vi "transfer char run_subvi_SMU4_14_05_22_JWa.vi"(0 "VISA session":refnum<visa-resource-name>="GPIB0::17::INSTR", 1 "Y2 axis settings":T5={"Y2 axis on/off"=FALSE, "MINIMUM"=0.0, "MAXIMUM"=1.0, "Variable name"="Ig", "LIN or LOG axis"="LIN"} {"MAXIMUM" format="%.9f"; "MINIMUM" format="%.9f"}, 3 "LKG Path":path, 5 "Var1 sweep settings":T7={"start"=40.0, "stop"=-40.0, "step (linear only)"=-1.0, "sweep spacing (linear: 0)"=0, "sweep mode"=FALSE, "compliance (V)"=100.0, "compliance (A)"=0.001} {"compliance (A)" format="%^.2e"; "compliance (V)" format="%.2f"; "sweep spacing (linear: 0)" items=["linear", "log 10", "log 25", "log 50"]; "step (linear only)" format="%.2f"; "stop" format="%.2f"; "start" format="%.2f"}, 7 "Var2 step settings":T6={"compliance (A)"=0.001, "compliance (V)"=100.0, "start"=-2.0, "total points"=2, "step"=-38.0} {"step" format="%.2f"; "start" format="%.2f"; "compliance (V)" format="%.2f"; "compliance (A)" format="%^.2e"}, 9 "integration time":u32(slide) scale=0.0..2.0, 11 "Input Path":path, 12 "Dielectric Constant":dbl=5.0, 13 "Sample Properties:":T4 {"Date Created" format="%<%x>T"}) -> (2 "Check Cluster":T2, 4 "Output":T3 {"Mobility-Lin" format="%#_4e"; "Mobility-Sat" format="%#_4e"}, 6 "Graph Cluster":T1, 15 "error?":errorcluster)   [LabVIEW 2012]
uses:
  <vilib>/Utility/file.llb/Write To Spreadsheet File (DBL).vi
panel:
  out "concatenated string":string
  in  "Output Path":path
  in  "Temp (K)":dbl=0.001 format="%^.2e"
  in  "NumPts":dbl=5.0
  out "Numeric":dbl
  out "min r":dbl
  out "max r":dbl
  out "error? 2":errorcluster
  in  "MAXIMUM":ext format="%.2e"
  in  "MINIMUM":ext=-1e-05 format="%_2e"
  out "Gate Current Plot":cluster{"trace":dbl[], "trace":dbl[]}(graph)
  in  "Y1 axis":string="Id"
  out "graphic display":cluster{"trace":dbl[], "trace":dbl[]}(graph)
  in  "wait time parameter":dbl=1.0
  in  "Value (Either V or A) 4":dbl
  in  "Value (Either V or A) 3":dbl
  in  "Value (Either V or A) 2":dbl
  in  "Value (V or A)":dbl
  in  "compliance (A)":dbl=0.001 format="%^.2e"
  in  "compliance (V)":dbl=100.0 format="%^.2e"
  in  "Iname":string="Is"
  in  "Vname":string="Vs"
  in  "Function":u16(ring)=4 items=["disabled", "Var1", "Var2", "Var1'", "Constant"]
  in  "Mode":u16(ring)=4 items=["V", "I", "VPulse", "IPulse", "Common"]
  in  "Iname 4":string="Ig"
  in  "Vname 4":string="Vg"
  in  "Function 4":u16(ring)=1 items=["disabled", "Var1", "Var2", "Var1'", "Constant"]
  in  "Mode 4":u16(ring) items=["V", "I", "VPulse", "IPulse", "Common"]
  in  "Iname 3":string="I3"
  in  "Vname 3":string="V3"
  in  "Function 3":u16(ring)=4 items=["disabled", "Var1", "Var2", "Var1'", "Constant"]
  in  "Mode 3":u16(ring) items=["V", "I", "VPulse", "IPulse", "Common"]
  in  "Iname 2":string="Id"
  in  "Vname 2":string="Vd"
  in  "Function 2":u16(ring)=2 items=["disabled", "Var1", "Var2", "Var1'", "Constant"]
  in  "Mode 2":u16(ring) items=["V", "I", "VPulse", "IPulse", "Common"]
  in  "reset":bool=TRUE
  # "SMU1"
  # "SMU2"
  # "SMU3"
  # "SMU4"
  # "Sample Properties:"
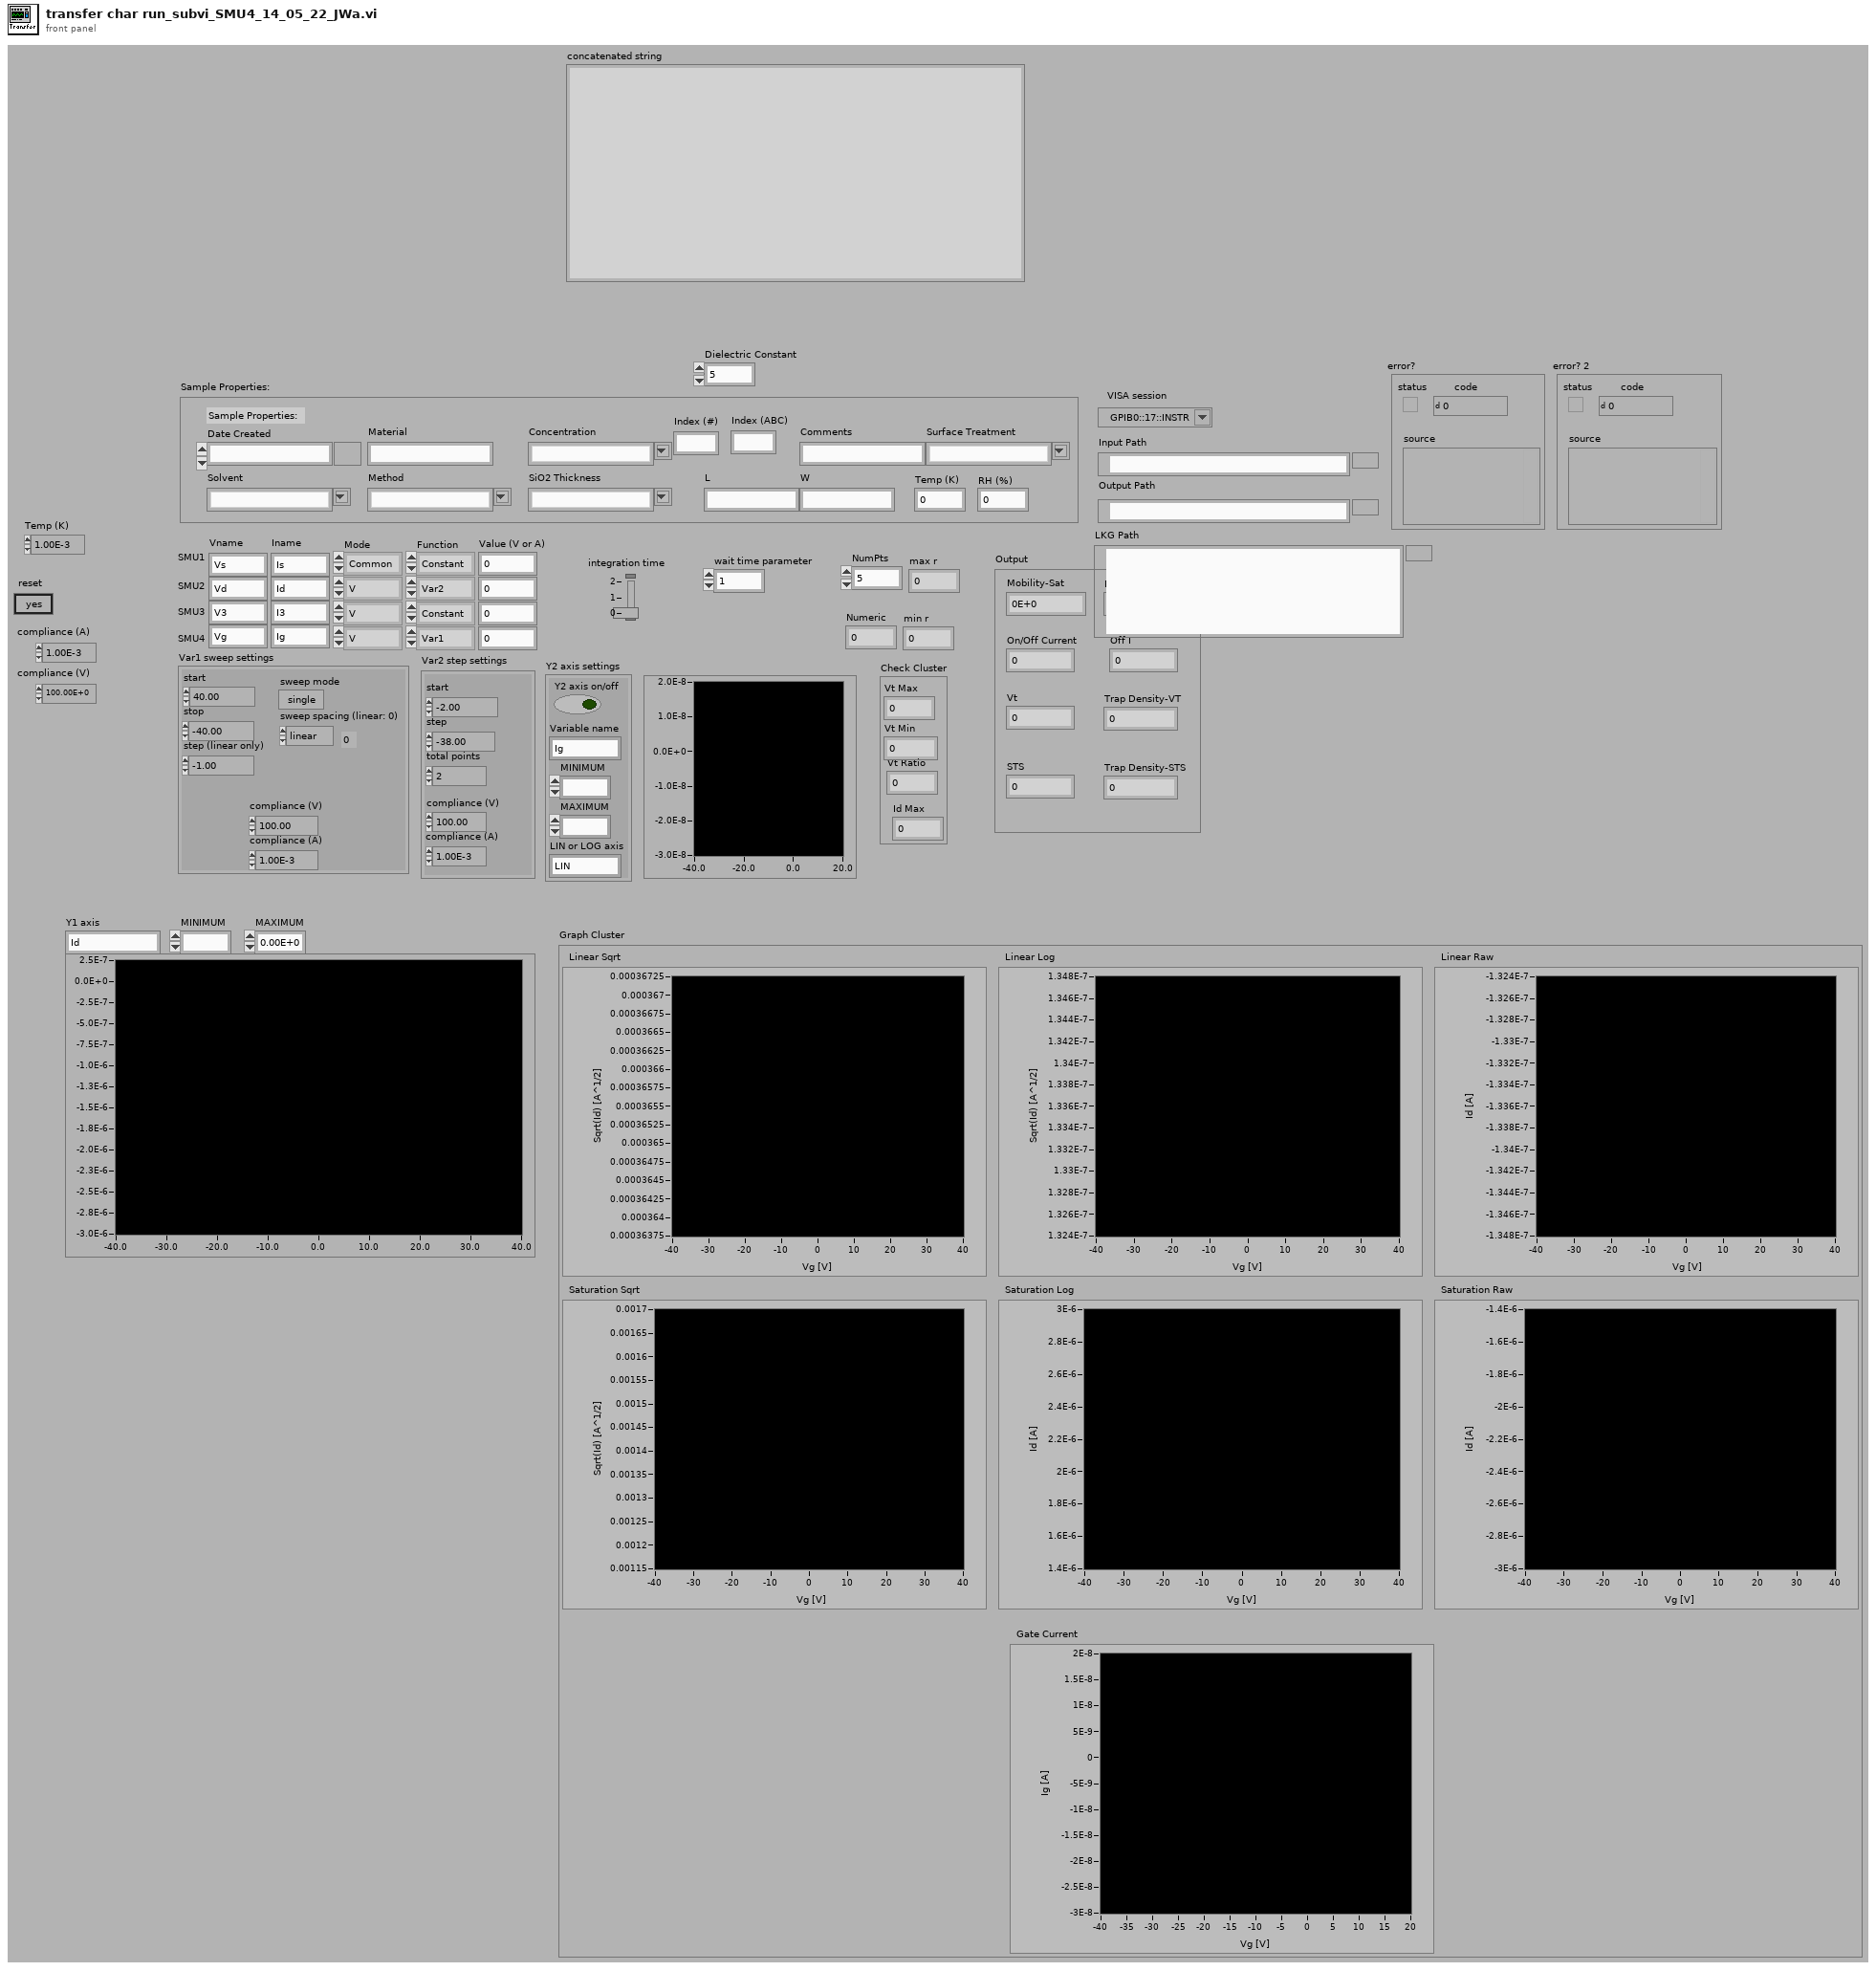
[diagram p1: front panel]
types:
  T1 = cluster{"Linear Sqrt":cluster{dbl[], "trace":dbl[]}[], "Linear Log":cluster{dbl[], "trace":dbl[]}[], "Linear Raw":cluster{dbl[], dbl[]}[], "Saturation Sqrt":cluster{dbl[], "trace":dbl[]}[], "Saturation Log":cluster{dbl[], "trace":dbl[]}[], "Saturation Raw":cluster{dbl[], "trace":dbl[]}[], "Gate Current":cluster{dbl[], "trace":dbl[]}[]}
  T2 = cluster{"Vt Max":i32, "Vt Min":i32, "Vt Ratio":i32, "Id Max":dbl}
  T3 = cluster{"Mobility-Sat":dbl, "Mobility-Lin":dbl, "On/Off Current":dbl, "Off I":dbl, "Vt":dbl, "STS":dbl, "Trap Density-VT":dbl, "Trap Density-STS":dbl}
  T4 = cluster{"Date Created":timestamp, "Material":string, "Solvent":string, "Concentration":string, "Method":string, "SiO2 Thickness":string, "Index (#)":string, "Index (ABC)":string, "L":string, "W":string, "Surface Treatment":string, "Comments":string, "Temp (K)":dbl, "RH (%)":dbl}
  T5 = cluster{"Y2 axis on/off":bool, "MINIMUM":ext, "MAXIMUM":ext, "Variable name":string, "LIN or LOG axis":string}
  T6 = cluster{"compliance (A)":dbl, "compliance (V)":dbl, "start":dbl, "total points":u16, "step":dbl}
  T7 = cluster{"start":dbl, "stop":dbl, "step (linear only)":dbl, "sweep spacing (linear: 0)":u16, "sweep mode":bool, "compliance (V)":dbl, "compliance (A)":dbl}
  T8 = cluster{"Vt Max":dbl, "Vt Min":dbl, "Vt Ratio":dbl, "Id Max":dbl}
  T9 = cluster{"Mobility-Sat":dbl, "Mobility-Lin":dbl, "On/Off I-Sat":dbl, "Off I-Sat":dbl, "VT-Sat":dbl, "Sub Threshold Swing":dbl, "Trap Density-VT":dbl, "Trap Density (N)":dbl}
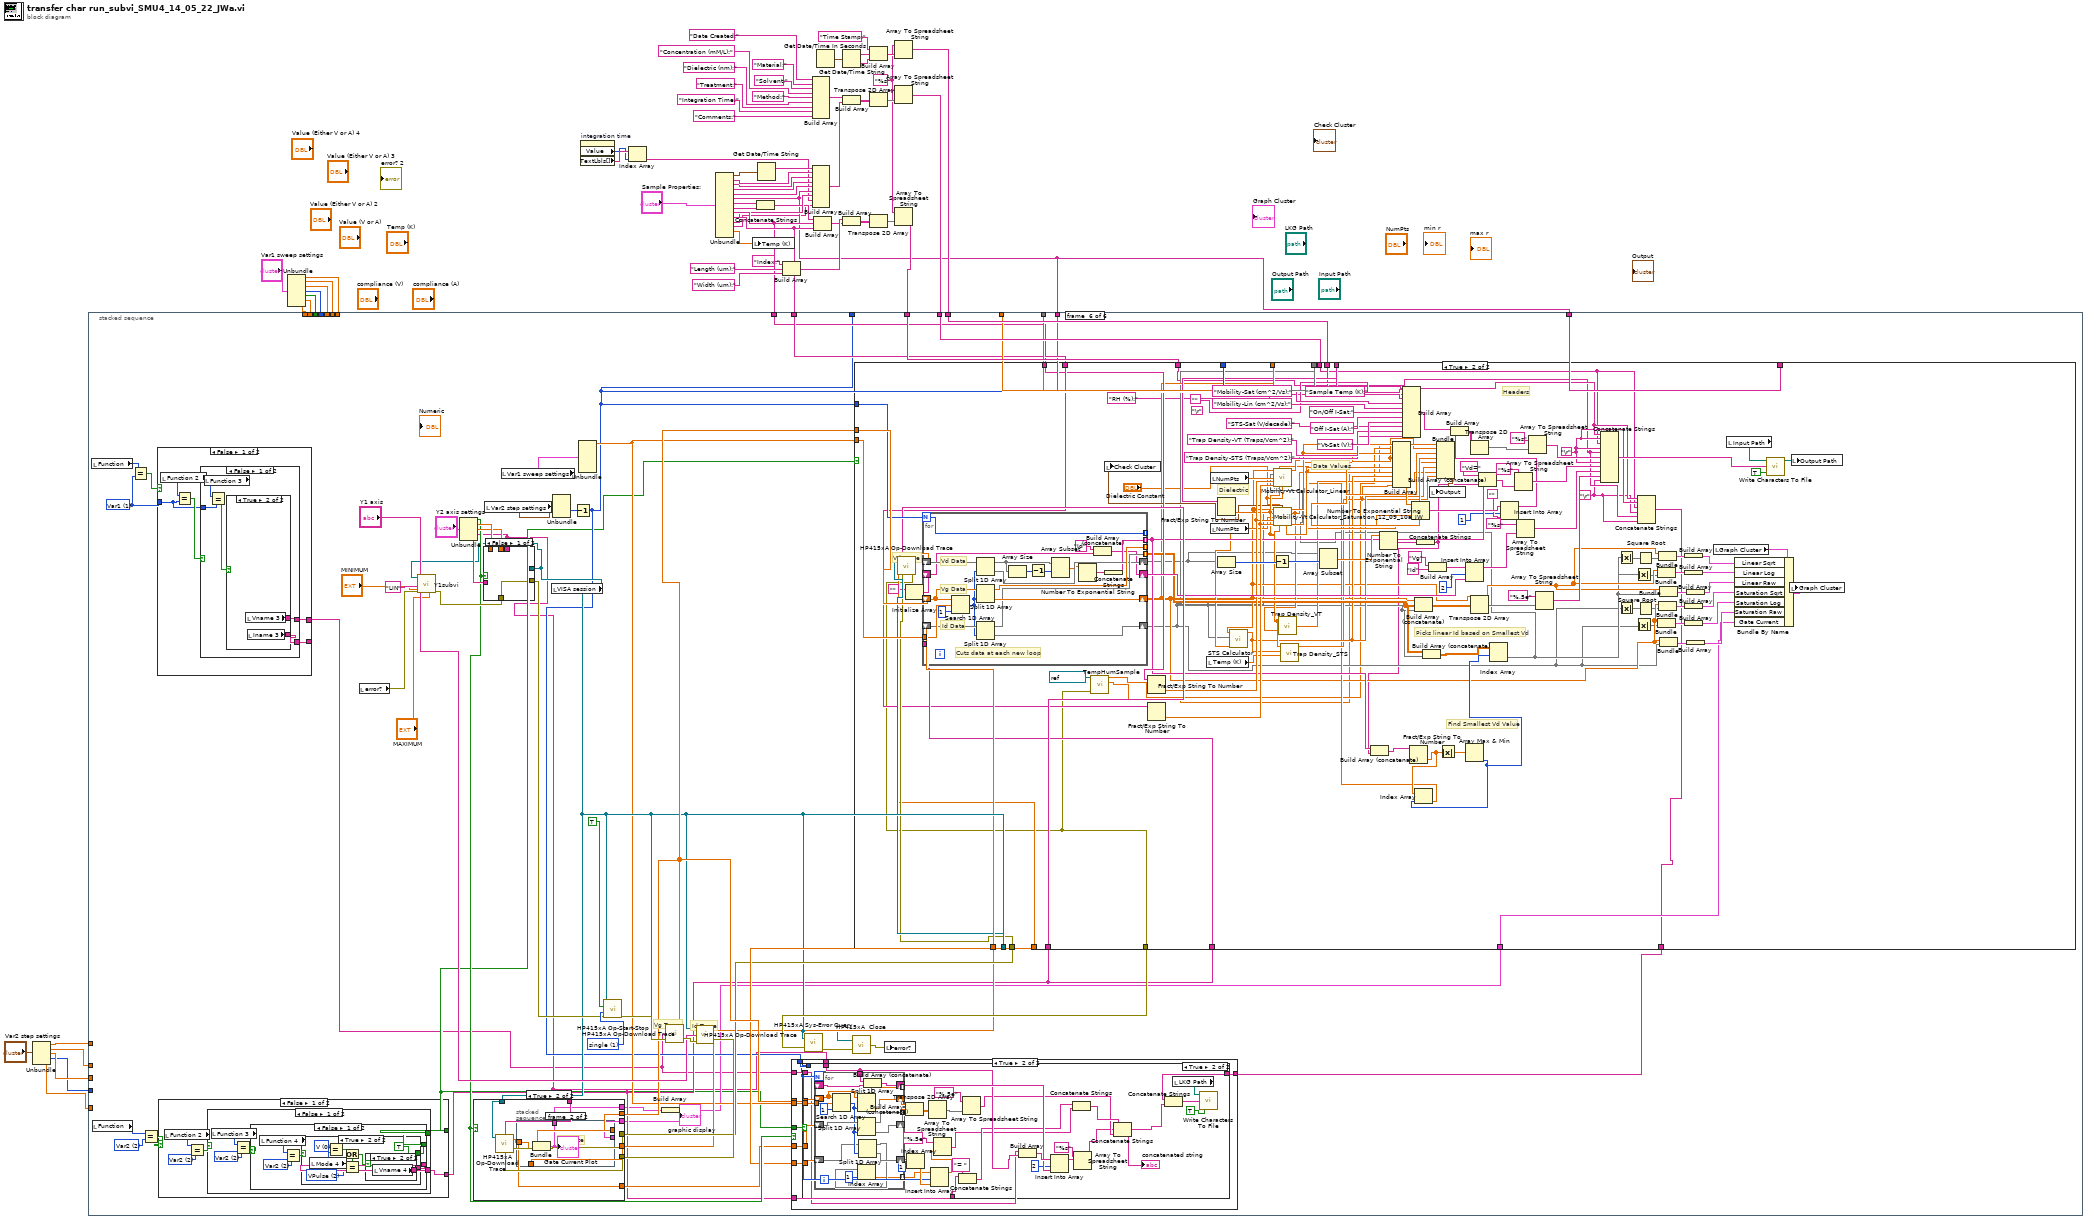
[diagram p0: block diagram]
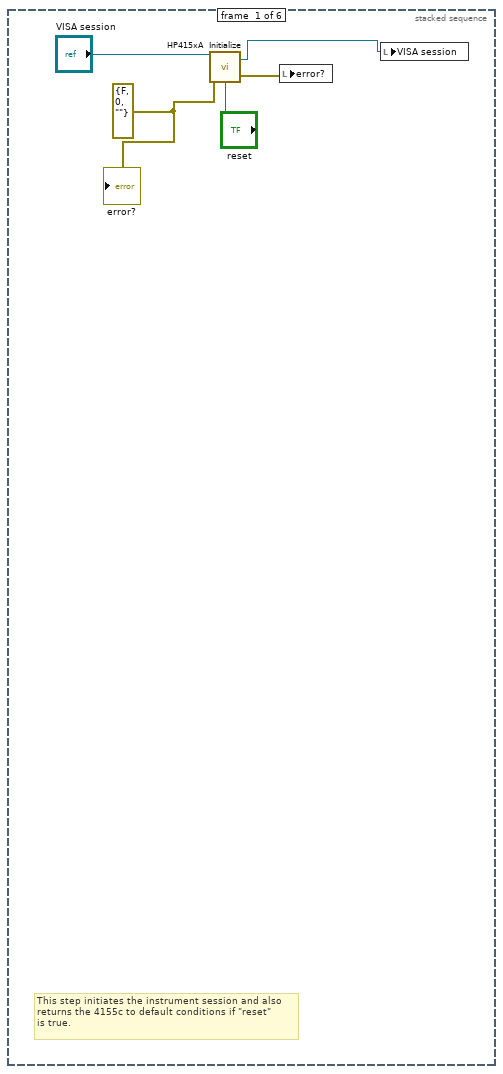
[diagram p2: hidden frame]
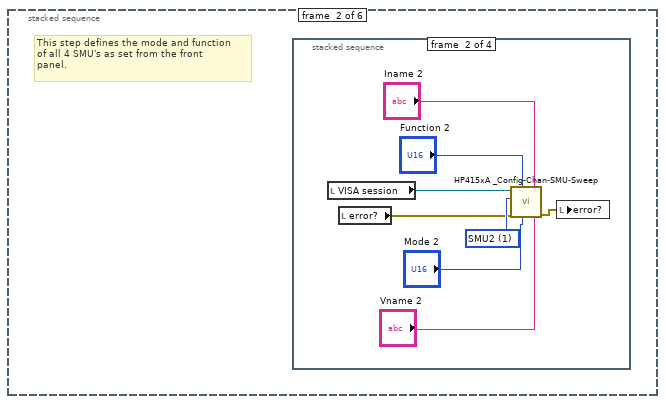
[diagram p3: hidden frame]
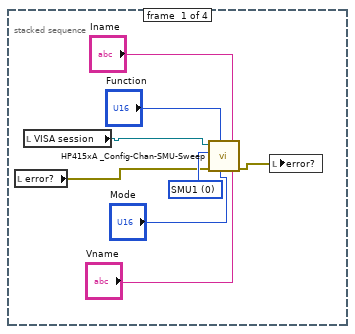
[diagram p4: hidden frame]
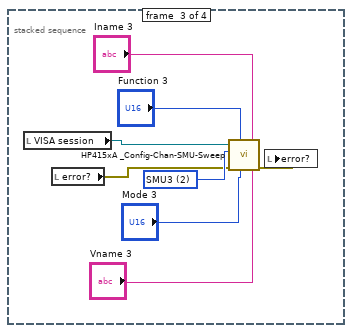
[diagram p5: hidden frame]
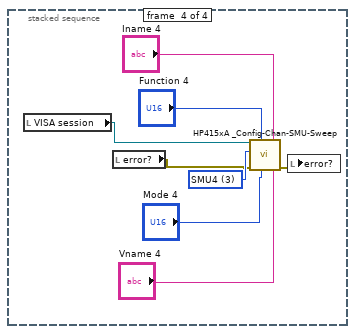
[diagram p6: hidden frame]
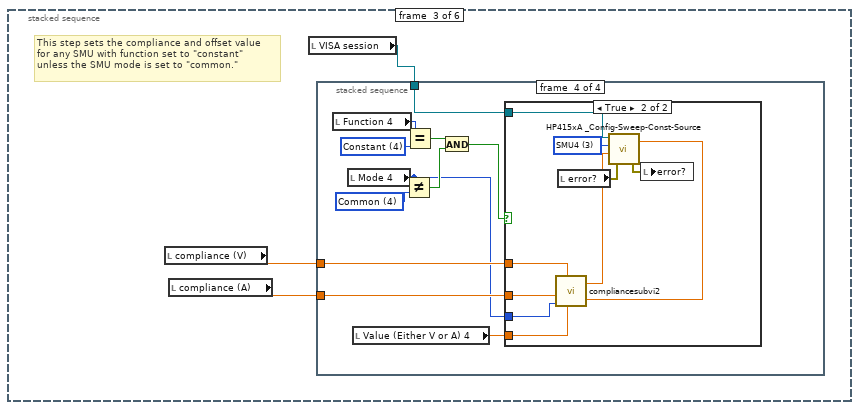
[diagram p7: hidden frame]
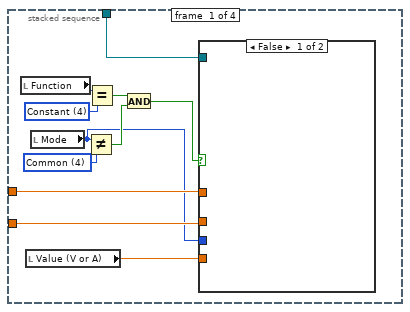
[diagram p8: hidden frame]
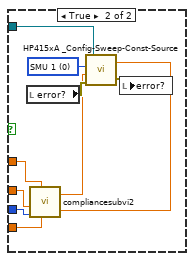
[diagram p9: hidden frame]
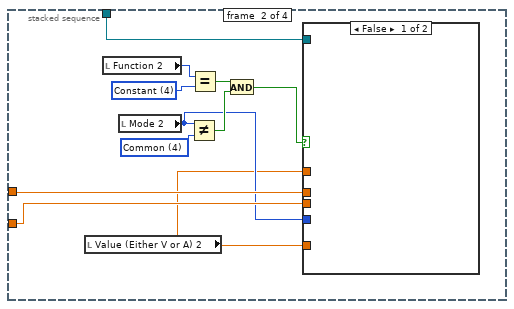
[diagram p10: hidden frame]
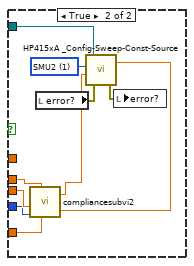
[diagram p11: hidden frame]
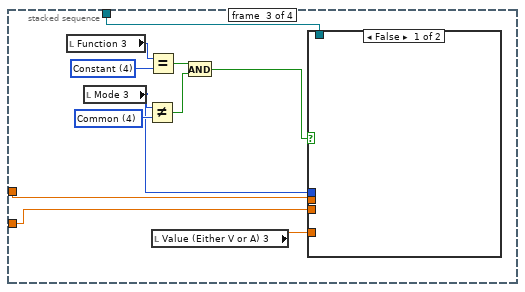
[diagram p12: hidden frame]
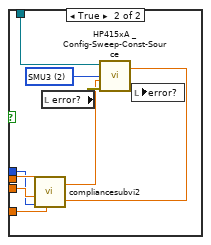
[diagram p13: hidden frame]
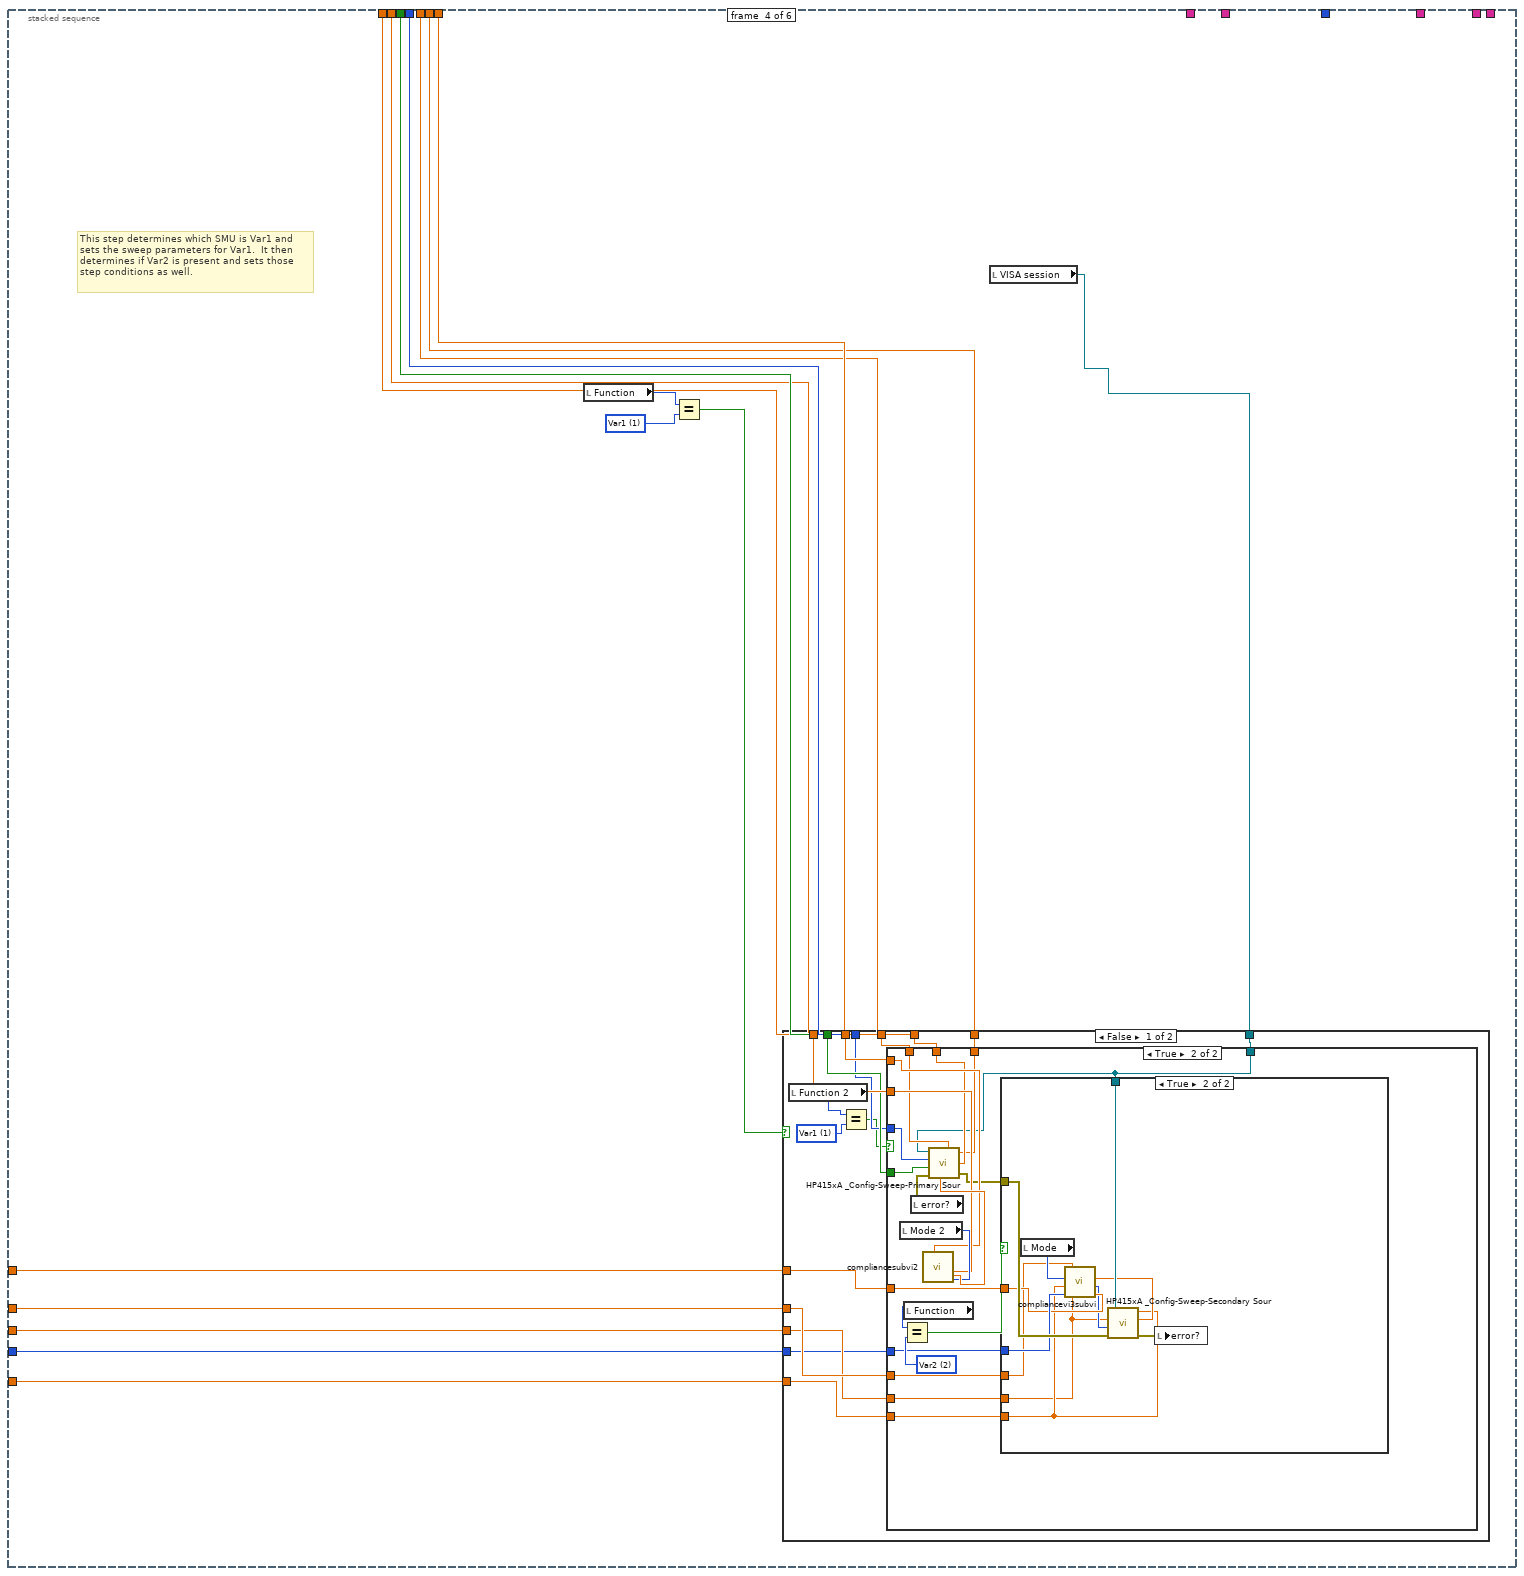
[diagram p15: hidden frame]
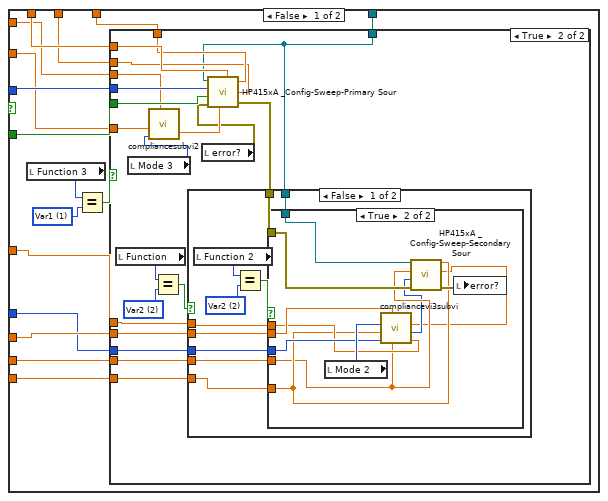
[diagram p16: hidden frame]
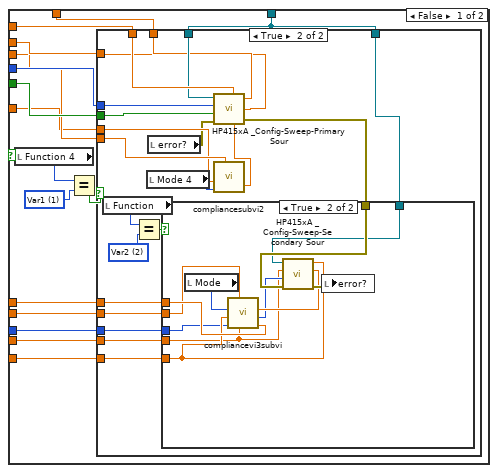
[diagram p17: hidden frame]
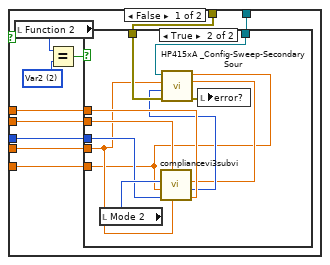
[diagram p19: hidden frame]
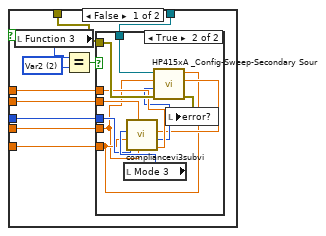
[diagram p20: hidden frame]
diagram:
  w7 = "%s"
  n1 = Unbundle("Var2 step settings") -> ("compliance (A)"=w53:dbl, "compliance (V)"=w52:dbl, "start"=w51:dbl, "total points"=w50:u16, "step"=w49:dbl)
  n2 = Unbundle("Var1 sweep settings") -> ("start"=w61:dbl, "stop"=w60:dbl, "step (linear only)"=w59:dbl, "sweep spacing (linear: 0)"=w58:u16, "sweep mode"=w57:bool, "compliance (V)"=w56:dbl, "compliance (A)"=w55:dbl)
  n3 = property on="integration time" class="Slide (strict)"() -> ("Value"=w2:u32, "TextLbls[]"=w3:string[])  [unwired: 2 in, 2 out]
  n4 = Index Array(array=w3, index=w2) -> (element=w1:string)
  n5 = Unbundle("Sample Properties:") -> ("Date Created"=w21:timestamp, "Material"=w20:string, "Solvent"=w17:string, "Concentration"=w16:string, "Method"=w19:string, "SiO2 Thickness"=w8:string, "Index (#)"=w12:string, "Index (ABC)"=w11:string, "L"=w14:string, "W"=w15:string, "Surface Treatment"=w13:string, "Comments"=w4:string, "Temp (K)"=w9:dbl)  [unwired: 1 out]
  n6 = local write "Temp (K)"(w9) -> ()
  n7 = Concatenate Strings(w12, w11) -> (w10:string)
  n8 = Get Date/Time String(seconds (now)=w21) -> (date string=w47:string)  [unwired: 2 in, 1 out]
  n9 = Build Array("Index:", "Length (um):", "Width (um):") -> (w27:string[])
  n10 = Build Array("Date Created:", "Material:", "Solvent:", "Concentration (mM/L):", "Method:", "Dielectric (nm):", "Treatment:", "Integration Time:", "Comments:") -> (w31:string[])
  n11 = Build Array(w47, w20, w17, w16, w19, w8, w13, w1, w4) -> (w30:string[])
  n12 = Build Array(w10, w14, w15) -> (w26:string[])
  n13 = Get Date/Time In Seconds() -> (seconds since 1Jan1904=w42:timestamp)
  n14 = Get Date/Time String(seconds (now)=w42) -> (date string=w41:string, time string=w40:string)  [unwired: 2 in]
  n15 = Build Array(w31, w30) -> (w29:string[][])
  n16 = Build Array(w27, w26) -> (w25:string[][])
  n17 = Build Array("Time Stamp:", w41, w40) -> (w39:string[])
  n18 = Transpose 2D Array(2D array=w29) -> (transposed array=w28:string[][])
  n19 = Transpose 2D Array(2D array=w25) -> (transposed array=w24:string[][])
  n20 = Array To Spreadsheet String(array=w39, 3:w7) -> (spreadsheet string=w32:string)  [unwired: 1 in]
  n21 = Array To Spreadsheet String(array=w28, 3:w7) -> (spreadsheet string=w35:string)  [unwired: 1 in]
  n22 = Array To Spreadsheet String(array=w24, 3:w7) -> (spreadsheet string=w23:string)  [unwired: 1 in]
  n23 = stacked-sequence {
    tunnel: w61 -> [_ _ _ w198 _ _]
    tunnel: w60 -> [_ _ _ w197 _ _]
    tunnel: w59 -> [_ _ _ w196 _ _]
    tunnel: w58 -> [_ _ _ w195 _ _]
    tunnel: w57 -> [_ _ _ w194 _ _]
    tunnel: w56 -> [_ _ _ w193 _ _]
    tunnel: w55 -> [_ _ _ w192 _ _]
    tunnel: w53 -> [_ _ _ w191 _ _]
    tunnel: w52 -> [_ _ _ w190 _ _]
    tunnel: w51 -> [_ _ _ w189 _ _]
    tunnel: w50 -> [_ _ _ w188 _ _]
    tunnel: w49 -> [_ _ _ w187 _ _]
    tunnel: w32 -> [_ _ _ _ _ w570]
    tunnel: w35 -> [_ _ _ _ _ w569]
    tunnel: w23 -> [_ _ _ _ _ w568]
    tunnel: [_ _ _ _ _ w567] -> _
    tunnel: [_ _ _ _ _ w566] -> _
    tunnel: [_ _ _ _ _ w563] -> _
    tunnel: w15 -> [_ _ _ _ _ w565]
    tunnel: w14 -> [_ _ _ _ _ w564]
    tunnel: w8 -> [_ _ _ _ _ w562]
    tunnel: w8 -> [_ _ _ _ _ w561]
    frame #0 {
      w66 = errorcluster {"status"=FALSE, "code"=0, "source"=""} ("error out")
      # "This step initiates the instrument session and also\nreturns the 4155c to default conditions if \"reset\"\nis true."
      n24 = call "HP415xA  Initialize.vi"("instrument descriptor"="VISA session", "reset"="reset", "error in (no error)"=w66) -> ("VISA session"=w63:refnum<visa-resource-name>, "error out"=w65:errorcluster)  [unwired: 2 in]
      n25 = local write "error?"(w65) -> ()
      n26 = local write "VISA session"(w63) -> ()
      "error?" <- w66
    }
    frame #1 {
      # "This step defines the mode and function\nof all 4 SMU's as set from the front\npanel."
      n27 = stacked-sequence {
        frame #0 {
          w75 = u32 0 items=["SMU1  ", "SMU2  ", "SMU3  ", "SMU4  ", "SMU5  ", "SMU6  "] ("unit to configure")
          n28 = local read "error?"() -> (w70:errorcluster)
          n29 = local read "VISA session"() -> (w68:refnum<visa-resource-name>)
          n30 = call "HP415xA _Config-Chan-SMU-Sweep.vi"("V name (max 6 chars)"="Vname", "I name (max 6 chars)"="Iname", "mode"="Mode", "function"="Function", "error in (no error)"=w70, "unit to configure"=w75, "VISA session"=w68) -> ("error out"=w69:errorcluster)  [unwired: 2 in]
          n31 = local write "error?"(w69) -> ()
        }
        frame #1 {
          w79 = u32 1 items=["SMU1  ", "SMU2  ", "SMU3  ", "SMU4  ", "SMU5  ", "SMU6  "] ("unit to configure")
          n32 = local read "VISA session"() -> (w76:refnum<visa-resource-name>)
          n33 = local read "error?"() -> (w77:errorcluster)
          n34 = call "HP415xA _Config-Chan-SMU-Sweep.vi"("V name (max 6 chars)"="Vname 2", "I name (max 6 chars)"="Iname 2", "mode"="Mode 2", "function"="Function 2", "error in (no error)"=w77, "unit to configure"=w79, "VISA session"=w76) -> ("error out"=w78:errorcluster)  [unwired: 2 in]
          n35 = local write "error?"(w78) -> ()
        }
        frame #2 {
          w87 = u32 2 items=["SMU1  ", "SMU2  ", "SMU3  ", "SMU4  ", "SMU5  ", "SMU6  "] ("unit to configure")
          n36 = local read "VISA session"() -> (w84:refnum<visa-resource-name>)
          n37 = local read "error?"() -> (w85:errorcluster)
          n38 = call "HP415xA _Config-Chan-SMU-Sweep.vi"("V name (max 6 chars)"="Vname 3", "I name (max 6 chars)"="Iname 3", "mode"="Mode 3", "function"="Function 3", "error in (no error)"=w85, "unit to configure"=w87, "VISA session"=w84) -> ("error out"=w86:errorcluster)  [unwired: 2 in]
          n39 = local write "error?"(w86) -> ()
        }
        frame #3 {
          w95 = u32 3 items=["SMU1  ", "SMU2  ", "SMU3  ", "SMU4  ", "SMU5  ", "SMU6  "] ("unit to configure")
          n40 = local read "VISA session"() -> (w92:refnum<visa-resource-name>)
          n41 = local read "error?"() -> (w94:errorcluster)
          n42 = call "HP415xA _Config-Chan-SMU-Sweep.vi"("V name (max 6 chars)"="Vname 4", "I name (max 6 chars)"="Iname 4", "mode"="Mode 4", "function"="Function 4", "error in (no error)"=w94, "unit to configure"=w95, "VISA session"=w92) -> ("error out"=w93:errorcluster)  [unwired: 2 in]
          n43 = local write "error?"(w93) -> ()
        }
      }
    }
    frame #2 {
      # "This step sets the compliance and offset value\nfor any SMU with function set to \"constant\"\nunless the SMU mode is set to \"common.\""
      n44 = local read "compliance (V)"() -> (w101:dbl)
      n45 = local read "compliance (A)"() -> (w102:dbl)
      n46 = local read "VISA session"() -> (w100:refnum<visa-resource-name>)
      n47 = stacked-sequence {
        tunnel: w100 -> [w111 w131 w150 w170]
        tunnel: w102 -> [w105 w127 w148 w168]
        tunnel: w101 -> [w104 w126 w147 w169]
        frame #0 {
          w109 = u16 4 items=["V", "I", "VPulse", "IPulse", "Common"] ("Mode")
          w113 = u16 4 items=["disabled", "Var1", "Var2", "Var1'", "Constant"] ("Function")
          n48 = local read "Function"() -> (w112:u16)
          n49 = local read "Value (V or A)"() -> (w106:dbl)
          n50 = local read "Mode"() -> (w103:u16)
          n51 = Not Equal?(x=w103, y=w109) -> (x != y?=w108:bool)
          n52 = Equal?(x=w112, y=w113) -> (x = y?=w110:bool)
          n53 = And(x=w110, y=w108) -> (x .and. y?=w107:bool)
          n54 = case shown="False" w107 {
            tunnel: w111 -> [_ w123]
            tunnel: w104 -> [_ w119]
            tunnel: w105 -> [_ w118]
            tunnel: w106 -> [_ w115]
            tunnel: w103 -> [_ w116]
            frame False {
            }
            frame True {
              w122 = u16 0 items=["SMU 1", "SMU2", "SMU3", "SMU4", "SMU5", "SMU6", "VSU1", "VSU2"] ("unit (SMU1:0)")
              n55 = local read "error?"() -> (w121:errorcluster)
              n56 = call "compliancesubvi2.vi"("Value1"=w115, "compliance (V)"=w119, "Mode"=w116, "compliance (A)"=w118) -> ("compliance"=w117:dbl, "constant"=w114:dbl)  [unwired: 2 in]
              n57 = call "HP415xA _Config-Sweep-Const-Source.vi"("compliance (SMUs only)"=w117, "error in (no error)"=w121, "source (V or A)"=w114, "unit (SMU1:0)"=w122, "VISA session"=w123) -> ("error out"=w120:errorcluster)
              n58 = local write "error?"(w120) -> ()
            }
          }
        }
        frame #1 {
          w128 = u16 4 items=["V", "I", "VPulse", "IPulse", "Common"] ("Mode 2")
          w129 = u16 4 items=["disabled", "Var1", "Var2", "Var1'", "Constant"] ("Function 2")
          n59 = local read "Value (Either V or A) 2"() -> (w124:dbl)
          n60 = local read "Function 2"() -> (w130:u16)
          n61 = local read "Mode 2"() -> (w125:u16)
          n62 = Not Equal?(x=w125, y=w128) -> (x != y?=w133:bool)
          n63 = Equal?(x=w130, y=w129) -> (x = y?=w134:bool)
          n64 = And(x=w134, y=w133) -> (x .and. y?=w132:bool)
          n65 = case shown="False" w132 {
            tunnel: w131 -> [_ w144]
            tunnel: w126 -> [_ w142]
            tunnel: w127 -> [_ w141]
            tunnel: w124 -> [_ _]
            tunnel: w125 -> [_ w137]
            tunnel: w124 -> [_ w136]
            frame False {
            }
            frame True {
              w143 = u16 1 items=["SMU 1", "SMU2", "SMU3", "SMU4", "SMU5", "SMU6", "VSU1", "VSU2"] ("unit (SMU1:0)")
              n66 = call "compliancesubvi2.vi"("Value1"=w136, "compliance (V)"=w142, "Mode"=w137, "compliance (A)"=w141) -> ("compliance"=w140:dbl, "constant"=w135:dbl)  [unwired: 2 in]
              n67 = local read "error?"() -> (w139:errorcluster)
              n68 = call "HP415xA _Config-Sweep-Const-Source.vi"("compliance (SMUs only)"=w140, "error in (no error)"=w139, "source (V or A)"=w135, "unit (SMU1:0)"=w143, "VISA session"=w144) -> ("error out"=w138:errorcluster)
              n69 = local write "error?"(w138) -> ()
            }
          }
        }
        frame #2 {
          w152 = u16 4 items=["V", "I", "VPulse", "IPulse", "Common"] ("Mode 2")
          w153 = u16 4 items=["disabled", "Var1", "Var2", "Var1'", "Constant"] ("Function 2")
          n70 = local read "Function 3"() -> (w151:u16)
          n71 = local read "Mode 3"() -> (w146:u16)
          n72 = Not Equal?(x=w146, y=w152) -> (x != y?=w154:bool)
          n73 = Equal?(x=w151, y=w153) -> (x = y?=w155:bool)
          n74 = local read "Value (Either V or A) 3"() -> (w149:dbl)
          n75 = And(x=w155, y=w154) -> (x .and. y?=w145:bool)
          n76 = case shown="False" w145 {
            tunnel: w150 -> [_ w163]
            tunnel: w149 -> [_ w157]
            tunnel: w148 -> [_ w160]
            tunnel: w147 -> [_ w159]
            tunnel: w146 -> [_ w158]
            frame False {
            }
            frame True {
              w162 = u16 2 items=["SMU 1", "SMU2", "SMU3", "SMU4", "SMU5", "SMU6", "VSU1", "VSU2"] ("unit (SMU1:0)")
              n77 = call "compliancesubvi2.vi"("Value1"=w157, "compliance (V)"=w159, "Mode"=w158, "compliance (A)"=w160) -> ("compliance"=w161:dbl, "constant"=w156:dbl)  [unwired: 2 in]
              n78 = local read "error?"() -> (w165:errorcluster)
              n79 = call "HP415xA _Config-Sweep-Const-Source.vi"("compliance (SMUs only)"=w161, "error in (no error)"=w165, "source (V or A)"=w156, "unit (SMU1:0)"=w162, "VISA session"=w163) -> ("error out"=w164:errorcluster)
              n80 = local write "error?"(w164) -> ()
            }
          }
        }
        frame #3 {
          w172 = u16 4 items=["V", "I", "VPulse", "IPulse", "Common"] ("Mode 4")
          w173 = u16 4 items=["disabled", "Var1", "Var2", "Var1'", "Constant"] ("Function 4")
          n81 = local read "Function 4"() -> (w174:u16)
          n82 = local read "Mode 4"() -> (w167:u16)
          n83 = local read "Value (Either V or A) 4"() -> (w166:dbl)
          n84 = Not Equal?(x=w167, y=w172) -> (x != y?=w175:bool)
          n85 = Equal?(x=w174, y=w173) -> (x = y?=w176:bool)
          n86 = And(x=w176, y=w175) -> (x .and. y?=w171:bool)
          n87 = case shown="True" w171 {
            tunnel: w170 -> [_ w185]
            tunnel: w169 -> [_ w181]
            tunnel: w168 -> [_ w182]
            tunnel: w167 -> [_ w180]
            tunnel: w166 -> [_ w179]
            frame False {
            }
            frame True {
              w186 = u16 3 items=["SMU 1", "SMU2", "SMU3", "SMU4", "SMU5", "SMU6", "VSU1", "VSU2"] ("unit (SMU1:0)")
              n88 = call "compliancesubvi2.vi"("Value1"=w179, "compliance (V)"=w181, "Mode"=w180, "compliance (A)"=w182) -> ("compliance"=w178:dbl, "constant"=w177:dbl)  [unwired: 2 in]
              n89 = local read "error?"() -> (w184:errorcluster)
              n90 = call "HP415xA _Config-Sweep-Const-Source.vi"("compliance (SMUs only)"=w178, "error in (no error)"=w184, "source (V or A)"=w177, "unit (SMU1:0)"=w186, "VISA session"=w185) -> ("error out"=w183:errorcluster)
              n91 = local write "error?"(w183) -> ()
            }
          }
        }
      }
    }
    frame #3 {
      w202 = u16 1 items=["disabled", "Var1", "Var2", "Var1'", "Constant"] ("Function")
      # "This step determines which SMU is Var1 and\nsets the sweep parameters for Var1.  It then\ndetermines if Var2 is present and sets those\nstep conditions as well."
      n92 = local read "Function"() -> (w201:u16)
      n93 = Equal?(x=w201, y=w202) -> (x = y?=w200:bool)
      n94 = local read "VISA session"() -> (w199:refnum<visa-resource-name>)
      n95 = case shown="False" w200 {
        tunnel: w193 -> [w215 w491]
        tunnel: w192 -> [w216 w490]
        tunnel: w195 -> [w213 w489]
        tunnel: w194 -> [w214 w488]
        tunnel: w196 -> [w210 w487]
        tunnel: w197 -> [w209 w486]
        tunnel: w198 -> [w211 w485]
        tunnel: w199 -> [w212 w474]
        tunnel: w191 -> [w207 w480]
        tunnel: w190 -> [w206 w479]
        tunnel: w189 -> [w205 w478]
        tunnel: w188 -> [w204 w477]
        tunnel: w187 -> [w203 w476]
        frame False {
          w218 = u16 1 items=["disabled", "Var1", "Var2", "Var1'", "Constant"] ("Function")
          n96 = local read "Function 2"() -> (w217:u16)
          n97 = Equal?(x=w217, y=w218) -> (x = y?=w208:bool)
          n98 = case shown="True" w208 {
            tunnel: w216 -> [w224 w417]
            tunnel: w215 -> [w225 w416]
            tunnel: w214 -> [w226 w415]
            tunnel: w213 -> [w227 w414]
            tunnel: w212 -> [w231 w403]
            tunnel: w211 -> [w230 w413]
            tunnel: w210 -> [w228 w412]
            tunnel: w209 -> [w229 w411]
            tunnel: w207 -> [w223 w406]
            tunnel: w206 -> [w222 w405]
            tunnel: w205 -> [w220 w404]
            tunnel: w204 -> [w221 w401]
            tunnel: w203 -> [w219 w400]
            frame False {
              w234 = u16 1 items=["disabled", "Var1", "Var2", "Var1'", "Constant"] ("Function")
              n99 = local read "Function 3"() -> (w233:u16)
              n100 = Equal?(x=w233, y=w234) -> (x = y?=w232:bool)
              n101 = case shown="True" w232 {
                tunnel: w231 -> [w235 w328]
                tunnel: w230 -> [w247 w345]
                tunnel: w229 -> [w244 w344]
                tunnel: w228 -> [w243 w343]
                tunnel: w227 -> [w246 w342]
                tunnel: w226 -> [w245 w341]
                tunnel: w225 -> [w242 w340]
                tunnel: w224 -> [w241 w339]
                tunnel: w223 -> [w240 w332]
                tunnel: w222 -> [w239 w331]
                tunnel: w221 -> [w238 w330]
                tunnel: w220 -> [w237 w327]
                tunnel: w219 -> [w236 w326]
                frame False {
                  w250 = u16 1 items=["disabled", "Var1", "Var2", "Var1'", "Constant"] ("Function")
                  n102 = local read "Function 4"() -> (w249:u16)
                  n103 = Equal?(x=w249, y=w250) -> (x = y?=w248:bool)
                  n104 = case shown="True" w248 {
                    tunnel: w247 -> [_ w269]
                    tunnel: w235 -> [_ w268]
                    tunnel: w246 -> [_ w267]
                    tunnel: w245 -> [_ w266]
                    tunnel: w244 -> [_ w265]
                    tunnel: w243 -> [_ w264]
                    tunnel: w242 -> [_ w263]
                    tunnel: w241 -> [_ w262]
                    tunnel: w240 -> [_ w257]
                    tunnel: w239 -> [_ w256]
                    tunnel: w238 -> [_ w255]
                    tunnel: w237 -> [_ w254]
                    tunnel: w236 -> [_ w253]
                    tunnel: w235 -> [_ w251]
                    frame False {
                    }
                    frame True {
                      w260 = u16 2 items=["disabled", "Var1", "Var2", "Var1'", "Constant"] ("Function")
                      n105 = local read "Function"() -> (w259:u16)
                      n106 = Equal?(x=w259, y=w260) -> (x = y?=w258:bool)
                      n107 = local read "Mode 4"() -> (w271:u16)
                      n108 = local read "error?"() -> (w261:errorcluster)
                      n109 = call "compliancesubvi2.vi"("compliance (V)"=w263, "Mode"=w271, "compliance (A)"=w262) -> ("compliance"=w270:dbl)  [unwired: 3 in, 1 out]
                      n110 = call "HP415xA _Config-Sweep-Primary Sour.vi"("step (linear only)"=w264, "stop"=w265, "start"=w269, "compliance"=w270, "error in (no error)"=w261, "sweep mode"=w266, "sweep spacing (linear: 0)"=w267, "VISA session"=w268) -> ("error out"=w252:errorcluster)  [unwired: 2 in]
                      n111 = case shown="True" w258 {
                        tunnel: w257 -> [w278 w321]
                        tunnel: w256 -> [w277 w316]
                        tunnel: w255 -> [w276 w315]
                        tunnel: w254 -> [w275 w317]
                        tunnel: w253 -> [w274 w320]
                        tunnel: w252 -> [w273 w323]
                        tunnel: w251 -> [w272 w322]
                        frame False {
                          w281 = u16 2 items=["disabled", "Var1", "Var2", "Var1'", "Constant"] ("Function")
                          n112 = local read "Function 2"() -> (w280:u16)
                          n113 = Equal?(x=w280, y=w281) -> (x = y?=w279:bool)
                          n114 = case shown="True" w279 {
                            tunnel: w278 -> [w289 w309]
                            tunnel: w277 -> [w288 w310]
                            tunnel: w276 -> [w287 w308]
                            tunnel: w275 -> [w286 w306]
                            tunnel: w274 -> [w285 w304]
                            tunnel: w273 -> [w284 w314]
                            tunnel: w272 -> [w282 w313]
                            frame False {
                              w291 = u16 2 items=["disabled", "Var1", "Var2", "Var1'", "Constant"] ("Function")
                              n115 = local read "Function 3"() -> (w283:u16)
                              n116 = Equal?(x=w283, y=w291) -> (x = y?=w290:bool)
                              n117 = case shown="True" w290 {
                                tunnel: w289 -> [_ w297]
                                tunnel: w288 -> [_ w298]
                                tunnel: w287 -> [_ w299]
                                tunnel: w286 -> [_ w293]
                                tunnel: w285 -> [_ w294]
                                tunnel: w284 -> [w292 w303]
                                tunnel: w282 -> [_ w302]
                                frame False {
                                n118 = local write "error?"(w292) -> ()
                                }
                                frame True {
                                n119 = local read "Mode 3"() -> (w301:u16)
                                n120 = call "compliancevi3subvi.vi"("compliance (A)"=w297, "start"=w293, "compliance (V)"=w298, "total points"=w299, "step"=w294, "Mode"=w301) -> ("total points 2"=w296:u16, "compliance"=w295:dbl)  [unwired: 1 in, 1 out]
                                n121 = call "HP415xA _Config-Sweep-Secondary Sour.vi"("compliance"=w295, "step"=w294, "error in (no error)"=w303, "total points"=w296, "start"=w293, "VISA session"=w302) -> ("error out"=w300:errorcluster)  [unwired: 1 in]
                                n122 = local write "error?"(w300) -> ()
                                }
                              }
                            }
                            frame True {
                              n123 = local read "Mode 2"() -> (w312:u16)
                              n124 = call "compliancevi3subvi.vi"("compliance (A)"=w309, "start"=w306, "compliance (V)"=w310, "total points"=w308, "step"=w304, "Mode"=w312) -> ("total points 2"=w307:u16, "compliance"=w305:dbl)  [unwired: 1 in, 1 out]
                              n125 = call "HP415xA _Config-Sweep-Secondary Sour.vi"("compliance"=w305, "step"=w304, "error in (no error)"=w314, "total points"=w307, "start"=w306, "VISA session"=w313) -> ("error out"=w311:errorcluster)  [unwired: 1 in]
                              n126 = local write "error?"(w311) -> ()
                            }
                          }
                        }
                        frame True {
                          n127 = local read "Mode"() -> (w325:u16)
                          n128 = call "compliancevi3subvi.vi"("compliance (A)"=w321, "start"=w317, "compliance (V)"=w316, "total points"=w315, "step"=w320, "Mode"=w325) -> ("total points 2"=w318:u16, "compliance"=w319:dbl)  [unwired: 1 in, 1 out]
                          n129 = call "HP415xA _Config-Sweep-Secondary Sour.vi"("compliance"=w319, "step"=w320, "error in (no error)"=w323, "total points"=w318, "start"=w317, "VISA session"=w322) -> ("error out"=w324:errorcluster)  [unwired: 1 in]
                          n130 = local write "error?"(w324) -> ()
                        }
                      }
                    }
                  }
                }
                frame True {
                  w335 = u16 2 items=["disabled", "Var1", "Var2", "Var1'", "Constant"] ("Function")
                  n131 = local read "Function"() -> (w334:u16)
                  n132 = local read "Mode 3"() -> (w337:u16)
                  n133 = call "compliancesubvi2.vi"("compliance (V)"=w340, "Mode"=w337, "compliance (A)"=w339) -> ("compliance"=w338:dbl)  [unwired: 3 in, 1 out]
                  n134 = Equal?(x=w334, y=w335) -> (x = y?=w333:bool)
                  n135 = local read "error?"() -> (w336:errorcluster)
                  n136 = call "HP415xA _Config-Sweep-Primary Sour.vi"("step (linear only)"=w343, "stop"=w344, "start"=w345, "compliance"=w338, "error in (no error)"=w336, "sweep mode"=w341, "sweep spacing (linear: 0)"=w342, "VISA session"=w328) -> ("error out"=w329:errorcluster)  [unwired: 2 in]
                  n137 = case shown="False" w333 {
                    tunnel: w332 -> [w350 w395]
                    tunnel: w331 -> [w349 w394]
                    tunnel: w330 -> [w347 w393]
                    tunnel: w329 -> [w352 w398]
                    tunnel: w328 -> [w351 w397]
                    tunnel: w327 -> [w346 w390]
                    tunnel: w326 -> [w348 w389]
                    frame False {
                      w355 = u16 2 items=["disabled", "Var1", "Var2", "Var1'", "Constant"] ("Function")
                      n138 = local read "Function 2"() -> (w354:u16)
                      n139 = Equal?(x=w354, y=w355) -> (x = y?=w353:bool)
                      n140 = case shown="True" w353 {
                        tunnel: w352 -> [w362 w387]
                        tunnel: w351 -> [w361 w386]
                        tunnel: w350 -> [w360 w382]
                        tunnel: w349 -> [w359 w383]
                        tunnel: w348 -> [w356 w381]
                        tunnel: w347 -> [w358 w384]
                        tunnel: w346 -> [w357 w380]
                        frame False {
                          w365 = u16 2 items=["disabled", "Var1", "Var2", "Var1'", "Constant"] ("Function")
                          n141 = local read "Function 4"() -> (w364:u16)
                          n142 = Equal?(x=w364, y=w365) -> (x = y?=w363:bool)
                          n143 = case shown="True" w363 {
                            tunnel: w362 -> [w366 w375]
                            tunnel: w361 -> [_ w376]
                            tunnel: w360 -> [_ w372]
                            tunnel: w359 -> [_ w373]
                            tunnel: w358 -> [_ w371]
                            tunnel: w357 -> [_ w368]
                            tunnel: w356 -> [_ w367]
                            frame False {
                              n144 = local write "error?"(w366) -> ()
                            }
                            frame True {
                              n145 = local read "Mode 4"() -> (w377:u16)
                              n146 = call "compliancevi3subvi.vi"("compliance (A)"=w372, "start"=w368, "compliance (V)"=w373, "total points"=w371, "step"=w367, "Mode"=w377) -> ("total points 2"=w370:u16, "compliance"=w369:dbl)  [unwired: 1 in, 1 out]
                              n147 = call "HP415xA _Config-Sweep-Secondary Sour.vi"("compliance"=w369, "step"=w367, "error in (no error)"=w375, "total points"=w370, "start"=w368, "VISA session"=w376) -> ("error out"=w374:errorcluster)  [unwired: 1 in]
                              n148 = local write "error?"(w374) -> ()
                            }
                          }
                        }
                        frame True {
                          n149 = local read "Mode 2"() -> (w388:u16)
                          n150 = call "compliancevi3subvi.vi"("compliance (A)"=w382, "start"=w380, "compliance (V)"=w383, "total points"=w384, "step"=w381, "Mode"=w388) -> ("total points 2"=w379:u16, "compliance"=w378:dbl)  [unwired: 1 in, 1 out]
                          n151 = call "HP415xA _Config-Sweep-Secondary Sour.vi"("compliance"=w378, "step"=w381, "error in (no error)"=w387, "total points"=w379, "start"=w380, "VISA session"=w386) -> ("error out"=w385:errorcluster)  [unwired: 1 in]
                          n152 = local write "error?"(w385) -> ()
                        }
                      }
                    }
                    frame True {
                      n153 = local read "Mode"() -> (w399:u16)
                      n154 = call "compliancevi3subvi.vi"("compliance (A)"=w395, "start"=w390, "compliance (V)"=w394, "total points"=w393, "step"=w389, "Mode"=w399) -> ("total points 2"=w392:u16, "compliance"=w391:dbl)  [unwired: 1 in, 1 out]
                      n155 = call "HP415xA _Config-Sweep-Secondary Sour.vi"("compliance"=w391, "step"=w389, "error in (no error)"=w398, "total points"=w392, "start"=w390, "VISA session"=w397) -> ("error out"=w396:errorcluster)  [unwired: 1 in]
                      n156 = local write "error?"(w396) -> ()
                    }
                  }
                }
              }
            }
            frame True {
              w409 = u16 2 items=["disabled", "Var1", "Var2", "Var1'", "Constant"] ("Function")
              n157 = local read "Mode 2"() -> (w418:u16)
              n158 = local read "Function"() -> (w408:u16)
              n159 = Equal?(x=w408, y=w409) -> (x = y?=w407:bool)
              n160 = local read "error?"() -> (w410:errorcluster)
              n161 = call "compliancesubvi2.vi"("compliance (V)"=w416, "Mode"=w418, "compliance (A)"=w417) -> ("compliance"=w419:dbl)  [unwired: 3 in, 1 out]
              n162 = call "HP415xA _Config-Sweep-Primary Sour.vi"("step (linear only)"=w412, "stop"=w411, "start"=w413, "compliance"=w419, "error in (no error)"=w410, "sweep mode"=w415, "sweep spacing (linear: 0)"=w414, "VISA session"=w403) -> ("error out"=w402:errorcluster)  [unwired: 2 in]
              n163 = case shown="True" w407 {
                tunnel: w406 -> [w425 w468]
                tunnel: w405 -> [w424 w467]
                tunnel: w404 -> [w422 w463]
                tunnel: w403 -> [w427 w473]
                tunnel: w402 -> [w421 w472]
                tunnel: w401 -> [w423 w469]
                tunnel: w400 -> [w420 w465]
                frame False {
                  w429 = u16 2 items=["disabled", "Var1", "Var2", "Var1'", "Constant"] ("Function")
                  n164 = local read "Function 3"() -> (w428:u16)
                  n165 = Equal?(x=w428, y=w429) -> (x = y?=w426:bool)
                  n166 = case shown="True" w426 {
                    tunnel: w427 -> [w435 w461]
                    tunnel: w425 -> [w434 w458]
                    tunnel: w424 -> [w432 w456]
                    tunnel: w423 -> [w433 w457]
                    tunnel: w422 -> [w430 w454]
                    tunnel: w421 -> [w436 w460]
                    tunnel: w420 -> [w431 w452]
                    frame False {
                      w439 = u16 2 items=["disabled", "Var1", "Var2", "Var1'", "Constant"] ("Function")
                      n167 = local read "Function 4"() -> (w438:u16)
                      n168 = Equal?(x=w438, y=w439) -> (x = y?=w437:bool)
                      n169 = case shown="True" w437 {
                        tunnel: w436 -> [w440 w451]
                        tunnel: w435 -> [_ w450]
                        tunnel: w434 -> [_ w447]
                        tunnel: w433 -> [_ w448]
                        tunnel: w432 -> [_ w446]
                        tunnel: w431 -> [_ w442]
                        tunnel: w430 -> [_ w443]
                        frame False {
                          n170 = local write "error?"(w440) -> ()
                        }
                        frame True {
                          n171 = local read "Mode 4"() -> (w445:u16)
                          n172 = call "compliancevi3subvi.vi"("compliance (A)"=w447, "start"=w443, "compliance (V)"=w446, "total points"=w448, "step"=w442, "Mode"=w445) -> ("total points 2"=w444:u16, "compliance"=w441:dbl)  [unwired: 1 in, 1 out]
                          n173 = call "HP415xA _Config-Sweep-Secondary Sour.vi"("compliance"=w441, "step"=w442, "error in (no error)"=w451, "total points"=w444, "start"=w443, "VISA session"=w450) -> ("error out"=w449:errorcluster)  [unwired: 1 in]
                          n174 = local write "error?"(w449) -> ()
                        }
                      }
                    }
                    frame True {
                      n175 = local read "Mode 3"() -> (w462:u16)
                      n176 = call "compliancevi3subvi.vi"("compliance (A)"=w458, "start"=w454, "compliance (V)"=w456, "total points"=w457, "step"=w452, "Mode"=w462) -> ("total points 2"=w455:u16, "compliance"=w453:dbl)  [unwired: 1 in, 1 out]
                      n177 = call "HP415xA _Config-Sweep-Secondary Sour.vi"("compliance"=w453, "step"=w452, "error in (no error)"=w460, "total points"=w455, "start"=w454, "VISA session"=w461) -> ("error out"=w459:errorcluster)  [unwired: 1 in]
                      n178 = local write "error?"(w459) -> ()
                    }
                  }
                }
                frame True {
                  n179 = local read "Mode"() -> (w470:u16)
                  n180 = call "compliancevi3subvi.vi"("compliance (A)"=w468, "start"=w463, "compliance (V)"=w467, "total points"=w469, "step"=w465, "Mode"=w470) -> ("total points 2"=w464:u16, "compliance"=w466:dbl)  [unwired: 1 in, 1 out]
                  n181 = call "HP415xA _Config-Sweep-Secondary Sour.vi"("compliance"=w466, "step"=w465, "error in (no error)"=w472, "total points"=w464, "start"=w463, "VISA session"=w473) -> ("error out"=w471:errorcluster)  [unwired: 1 in]
                  n182 = local write "error?"(w471) -> ()
                }
              }
            }
          }
        }
        frame True {
          w482 = u16 2 items=["disabled", "Var1", "Var2", "Var1'", "Constant"] ("Function 2")
          n183 = local read "error?"() -> (w484:errorcluster)
          n184 = local read "Mode"() -> (w492:u16)
          n185 = local read "Function 2"() -> (w483:u16)
          n186 = call "compliancesubvi2.vi"("compliance (V)"=w491, "Mode"=w492, "compliance (A)"=w490) -> ("compliance"=w493:dbl)  [unwired: 3 in, 1 out]
          n187 = call "HP415xA _Config-Sweep-Primary Sour.vi"("step (linear only)"=w487, "stop"=w486, "start"=w485, "compliance"=w493, "error in (no error)"=w484, "sweep mode"=w488, "sweep spacing (linear: 0)"=w489, "VISA session"=w474) -> ("error out"=w475:errorcluster)  [unwired: 2 in]
          n188 = Equal?(x=w483, y=w482) -> (x = y?=w481:bool)
          n189 = case shown="True" w481 {
            tunnel: w480 -> [w499 w543]
            tunnel: w479 -> [w500 w542]
            tunnel: w478 -> [w497 w539]
            tunnel: w477 -> [w498 w541]
            tunnel: w476 -> [w496 w537]
            tunnel: w475 -> [w495 w546]
            tunnel: w474 -> [w494 w544]
            frame False {
              w503 = u16 2 items=["disabled", "Var1", "Var2", "Var1'", "Constant"] ("Function 2")
              n190 = local read "Function 3"() -> (w502:u16)
              n191 = Equal?(x=w502, y=w503) -> (x = y?=w501:bool)
              n192 = case shown="True" w501 {
                tunnel: w500 -> [w508 w526]
                tunnel: w499 -> [w509 w527]
                tunnel: w498 -> [w506 w532]
                tunnel: w497 -> [w507 w529]
                tunnel: w496 -> [w505 w528]
                tunnel: w495 -> [w510 w535]
                tunnel: w494 -> [w504 w533]
                frame False {
                  w513 = u16 2 items=["disabled", "Var1", "Var2", "Var1'", "Constant"] ("Function 2")
                  n193 = local read "Function 4"() -> (w512:u16)
                  n194 = Equal?(x=w512, y=w513) -> (x = y?=w511:bool)
                  n195 = case shown="True" w511 {
                    tunnel: w510 -> [w514 w525]
                    tunnel: w509 -> [_ w515]
                    tunnel: w508 -> [_ w516]
                    tunnel: w507 -> [_ w517]
                    tunnel: w506 -> [_ w522]
                    tunnel: w505 -> [_ w519]
                    tunnel: w504 -> [_ w523]
                    frame False {
                      n196 = local write "error?"(w514) -> ()
                    }
                    frame True {
                      n197 = local read "Mode 4"() -> (w521:u16)
                      n198 = call "compliancevi3subvi.vi"("compliance (A)"=w515, "start"=w517, "compliance (V)"=w516, "total points"=w522, "step"=w519, "Mode"=w521) -> ("total points 2"=w518:u16, "compliance"=w520:dbl)  [unwired: 1 in, 1 out]
                      n199 = call "HP415xA _Config-Sweep-Secondary Sour.vi"("compliance"=w520, "step"=w519, "error in (no error)"=w525, "total points"=w518, "start"=w517, "VISA session"=w523) -> ("error out"=w524:errorcluster)  [unwired: 1 in]
                      n200 = local write "error?"(w524) -> ()
                    }
                  }
                }
                frame True {
                  n201 = local read "Mode 3"() -> (w536:u16)
                  n202 = call "compliancevi3subvi.vi"("compliance (A)"=w527, "start"=w529, "compliance (V)"=w526, "total points"=w532, "step"=w528, "Mode"=w536) -> ("total points 2"=w531:u16, "compliance"=w530:dbl)  [unwired: 1 in, 1 out]
                  n203 = call "HP415xA _Config-Sweep-Secondary Sour.vi"("compliance"=w530, "step"=w528, "error in (no error)"=w535, "total points"=w531, "start"=w529, "VISA session"=w533) -> ("error out"=w534:errorcluster)  [unwired: 1 in]
                  n204 = local write "error?"(w534) -> ()
                }
              }
            }
            frame True {
              n205 = local read "Mode 2"() -> (w547:u16)
              n206 = call "compliancevi3subvi.vi"("compliance (A)"=w543, "start"=w539, "compliance (V)"=w542, "total points"=w541, "step"=w537, "Mode"=w547) -> ("total points 2"=w540:u16, "compliance"=w538:dbl)  [unwired: 1 in, 1 out]
              n207 = call "HP415xA _Config-Sweep-Secondary Sour.vi"("compliance"=w538, "step"=w537, "error in (no error)"=w546, "total points"=w540, "start"=w539, "VISA session"=w544) -> ("error out"=w545:errorcluster)  [unwired: 1 in]
              n208 = local write "error?"(w545) -> ()
            }
          }
        }
      }
    }
    frame #4 {
      # "This step sets the integration time."
      n209 = local read "VISA session"() -> (w548:refnum<visa-resource-name>)
      n210 = local read "error?"() -> (w552:errorcluster)
      n211 = call "HP415xA _Config-Meas-Timing.vi"("error in (no error)"=w552, "wait time parameter"="wait time parameter", "integration time"="integration time", "VISA session"=w548) -> ("error out"=w551:errorcluster)  [unwired: 2 in]
      n212 = local write "error?"(w551) -> ()
    }
    frame #5 {
      w593 = u32 1 items=["stop  ", "single  ", "single-append  ", "stress start  ", "continuous  ", "standby on  ", "standby off  ", "zero  "] ("function (stop:0)")
      w597 = u16 2 items=["disabled", "Var1", "Var2", "Var1'", "Constant"] ("Function")
      w601 = u16 1 items=["disabled", "Var1", "Var2", "Var1'", "Constant"] ("Function")
      # "Id Trace"
      # "Vg Trace"
      n213 = local read "Function"() -> (w603:u16)
      n214 = local read "Function"() -> (w596:u16)
      n215 = Equal?(x=w603, y=w601) -> (x = y?=w602:bool)
      n216 = Equal?(x=w596, y=w597) -> (x = y?=w595:bool)
      n217 = case shown="False" w602 {
        tunnel: [w911 w926] -> w554
        tunnel: [w912 w925] -> _
        tunnel: w601 -> [w909 _]
        frame False {
          n218 = local read "Function 2"() -> (w913:u16)
          n219 = Equal?(x=w913, y=w909) -> (x = y?=w910:bool)
          n220 = case shown="False" w910 {
            tunnel: [w914 w924] -> w912
            tunnel: [w915 w923] -> w911
            tunnel: w909 -> [w918 _]
            frame False {
              n221 = local read "Function 3"() -> (w917:u16)
              n222 = Equal?(x=w917, y=w918) -> (x = y?=w916:bool)
              n223 = case shown="True" w916 {
                tunnel: [w920 w922] -> w915
                tunnel: [w919 w921] -> w914
                frame False {
                  n224 = local read "Vname 4"() -> (w920:string)
                  n225 = local read "Iname 4"() -> (w919:string)
                }
                frame True {
                  n226 = local read "Vname 3"() -> (w922:string)
                  n227 = local read "Iname 3"() -> (w921:string)
                }
              }
            }
            frame True {
              n228 = local read "Iname 2"() -> (w924:string)
              n229 = local read "Vname 2"() -> (w923:string)
            }
          }
        }
        frame True {
          n230 = local read "Vname"() -> (w926:string)
          n231 = local read "Iname"() -> (w925:string)
        }
      }
      n232 = case shown="False" w595 {
        tunnel: [w853 w906] -> w560
        tunnel: [w852 TRUE ("x = y?")] -> w556
        frame False {
          w856 = u16 2 items=["disabled", "Var1", "Var2", "Var1'", "Constant"] ("Function")
          n233 = local read "Function 2"() -> (w855:u16)
          n234 = Equal?(x=w855, y=w856) -> (x = y?=w854:bool)
          n235 = case shown="False" w854 {
            tunnel: [w858 w896] -> w853
            tunnel: [w857 TRUE ("x = y?")] -> w852
            frame False {
              w861 = u16 2 items=["disabled", "Var1", "Var2", "Var1'", "Constant"] ("Function")
              n236 = local read "Function 3"() -> (w860:u16)
              n237 = Equal?(x=w860, y=w861) -> (x = y?=w859:bool)
              n238 = case shown="False" w859 {
                tunnel: [w866 w886] -> w858
                tunnel: [w862 TRUE ("x = y?")] -> w857
                frame False {
                  w865 = u16 2 items=["disabled", "Var1", "Var2", "Var1'", "Constant"] ("Function")
                  n239 = local read "Function 4"() -> (w864:u16)
                  n240 = Equal?(x=w864, y=w865) -> (x = y?=w863:bool)
                  n241 = case shown="True" w863 {
                    tunnel: ["0" ("Vname 4") w876] -> w866
                    tunnel: [FALSE ("x = y?") TRUE ("x = y?")] -> w862
                    frame False {
                    }
                    frame True {
                      w870 = u16 2 items=["V", "I", "VPulse", "IPulse", "Common"] ("Mode 2")
                      w873 = u16 0 items=["V", "I", "VPulse", "IPulse", "Common"] ("Mode 2")
                      n242 = local read "Mode 4"() -> (w872:u16)
                      n243 = Equal?(x=w873, y=w872) -> (x = y?=w874:bool)
                      n244 = Equal?(x=w872, y=w870) -> (x = y?=w871:bool)
                      n245 = Or(x=w874, y=w871) -> (x .or. y?=w869:bool)
                      n246 = case shown="True" w869 {
                        tunnel: [w877 w878] -> w876
                        frame False {
                          n247 = local read "Iname 4"() -> (w877:string)
                        }
                        frame True {
                          n248 = local read "Vname 4"() -> (w878:string)
                        }
                      }
                    }
                  }
                }
                frame True {
                  w882 = u16 2 items=["V", "I", "VPulse", "IPulse", "Common"] ("Mode 2")
                  w881 = u16 0 items=["V", "I", "VPulse", "IPulse", "Common"] ("Mode 2")
                  n249 = local read "Mode 3"() -> (w880:u16)
                  n250 = Equal?(x=w881, y=w880) -> (x = y?=w884:bool)
                  n251 = Equal?(x=w880, y=w882) -> (x = y?=w883:bool)
                  n252 = Or(x=w884, y=w883) -> (x .or. y?=w879:bool)
                  n253 = case shown="False" w879 {
                    tunnel: [w887 w888] -> w886
                    frame False {
                      n254 = local read "Iname 3"() -> (w887:string)
                    }
                    frame True {
                      n255 = local read "Vname 3"() -> (w888:string)
                    }
                  }
                }
              }
            }
            frame True {
              w890 = u16 2 items=["V", "I", "VPulse", "IPulse", "Common"] ("Mode 2")
              w891 = u16 0 items=["V", "I", "VPulse", "IPulse", "Common"] ("Mode 2")
              n256 = local read "Mode 2"() -> (w892:u16)
              n257 = Equal?(x=w891, y=w892) -> (x = y?=w894:bool)
              n258 = Equal?(x=w892, y=w890) -> (x = y?=w893:bool)
              n259 = Or(x=w894, y=w893) -> (x .or. y?=w889:bool)
              n260 = case shown="True" w889 {
                tunnel: [w897 w898] -> w896
                frame False {
                  n261 = local read "Iname 2"() -> (w897:string)
                }
                frame True {
                  n262 = local read "Vname 2"() -> (w898:string)
                }
              }
            }
          }
        }
        frame True {
          w903 = u16 2 items=["V", "I", "VPulse", "IPulse", "Common"] ("Mode")
          w904 = u16 0 items=["V", "I", "VPulse", "IPulse", "Common"] ("Mode")
          n263 = local read "Mode"() -> (w902:u16)
          n264 = Equal?(x=w902, y=w904) -> (x = y?=w901:bool)
          n265 = Equal?(x=w902, y=w903) -> (x = y?=w900:bool)
          n266 = Or(x=w901, y=w900) -> (x .or. y?=w899:bool)
          n267 = case shown="True" w899 {
            tunnel: [w907 w908] -> w906
            frame False {
              n268 = local read "Iname"() -> (w907:string)
            }
            frame True {
              n269 = local read "Vname"() -> (w908:string)
            }
          }
        }
      }
      n270 = local read "error?"() -> (w585:errorcluster)
      n271 = Unbundle("Y2 axis settings") -> ("Y2 axis on/off"=w579:bool, "MINIMUM"=w590:ext, "MAXIMUM"=w589:ext, "Variable name"=w555:string, "LIN or LOG axis"=w588:string)
      n272 = local read "Var2 step settings"() -> (w599:T6)
      n273 = local read "Var1 sweep settings"() -> (w600:T7)
      n274 = local read "VISA session"() -> (w572:refnum<visa-resource-name>)
      n275 = call "Y1subvi.vi"("MAXIMUM"="MAXIMUM", "MINIMUM"="MINIMUM", "error in (no error)"=w585, "LIN or LOG axis"="LIN", "Variable name"="Y1 axis", "VISA In"=w572) -> ("error out"=w586:errorcluster)  [unwired: 4 in, 1 out]
      n276 = case shown="False" w579 {
        tunnel: w586 -> [w844 w851]
        tunnel: w572 -> [_ w850]
        tunnel: w590 -> [_ w849]
        tunnel: w589 -> [_ w848]
        tunnel: w555 -> [_ w847]
        tunnel: w588 -> [_ w846]
        tunnel: [w844 w845] -> w587
        frame False {
        }
        frame True {
          n277 = call "Y2subvi.vi"("MAXIMUM"=w848, "Variable name"=w847, "error in (no error)"=w851, "MINIMUM"=w849, "LIN or LOG axis"=w846, "VISA resource name"=w850) -> ("error out"=w845:errorcluster)
        }
      }
      n278 = Unbundle(w599) -> ("total points"=w598:u16)  [unwired: 4 out]
      n279 = Decrement(x=w598) -> (x-1=w563:u16)
      n280 = Unbundle(w600) -> ("start"=w571:dbl)  [unwired: 6 out]
      n281 = call "HP415xA Op-Start-Stop.vi"("error in (no error)"=w587, "function (stop:0)"=w593, "wait until finish"=TRUE, "VISA session"=w572) -> ("error out"=w592:errorcluster)  [unwired: 6 in, 1 out]
      n282 = call "HP415xA Op-Download Trace.vi"("error in (no error)"=w592, "trace (variable) name"=w554, "VISA session"=w572) -> ("error out"=w606:errorcluster, "trace"=w577:dbl[])
      n283 = call "HP415xA Op-Download Trace.vi"("error in (no error)"=w606, "trace (variable) name"="Y1 axis", "VISA session"=w572) -> ("error out"=w582:errorcluster, "trace"=w573:dbl[])
      n284 = case shown="True" w579 {
        tunnel: w582 -> [w828 w837]
        tunnel: w572 -> [_ w836]
        tunnel: w555 -> [_ w835]
        tunnel: [w828 w834] -> w574
        tunnel: w577 -> [w826 w833]
        tunnel: w573 -> [w827 w832]
        tunnel: [w825 w831] -> w559
        tunnel: [dbl[] [] ("trace") w830] -> w578
        tunnel: [cluster{"trace":dbl[], "trace":dbl[]} {"trace"=[], "trace"=[]} w829] -> w557
        frame False {
          n285 = Bundle("trace"=w826, "trace"=w827) -> (w825:cluster{"trace":dbl[], "trace":dbl[]})  [unwired: 1 in]
        }
        frame True {
          n286 = call "HP415xA Op-Download Trace.vi"("error in (no error)"=w837, "trace (variable) name"=w835, "VISA session"=w836) -> ("error out"=w834:errorcluster, "trace"=w830:dbl[])
          n287 = stacked-sequence {
            tunnel: w830 -> [_ w843]
            tunnel: w833 -> [w840 w842]
            tunnel: w832 -> [w839 _]
            tunnel: [w838 _] -> w831
            tunnel: [_ w841] -> w829
            frame #0 {
              n288 = Bundle("trace"=w840, "trace"=w839) -> (w838:cluster{"trace":dbl[], "trace":dbl[]})  [unwired: 1 in]
            }
            frame #1 {
              # "Ig Trace"
              n289 = Bundle("trace"=w842, "trace"=w843) -> (w841:cluster{"trace":dbl[], "trace":dbl[]})  [unwired: 1 in]
              "Gate Current Plot" <- w841
            }
          }
        }
      }
      "graphic display" <- w559
      n290 = Build Array(w557) -> (w558:cluster{"trace":dbl[], "trace":dbl[]}[])
      n291 = case shown="True" w556 {
        tunnel: w571 -> [_ w733]
        tunnel: w573 -> [w611 w732]
        tunnel: w577 -> [w612 w731]
        tunnel: w563 -> [_ w730]
        tunnel: w572 -> [_ w726]
        tunnel: w574 -> [_ w725]
        tunnel: [w613 w617] -> w576
        tunnel: w560 -> [_ w724]
        tunnel: w560 -> [_ w719]
        tunnel: [dbl[] [] ("trace") w723] -> w575
        tunnel: w570 -> [_ w627]
        tunnel: w569 -> [_ w619]
        tunnel: w568 -> [_ w625]
        tunnel: [_ w636] -> w567
        tunnel: [_ w631] -> w566
        tunnel: w565 -> [_ w702]
        tunnel: w564 -> [_ w701]
        tunnel: w563 -> [_ _]
        tunnel: w562 -> [_ _]
        tunnel: w561 -> [_ w685]
        tunnel: w558 -> [_ w628]
        tunnel: [_ w621] -> w553
        frame False {
          n292 = Build Array(w612, w611) -> (w608:dbl[][])
          n293 = local read "error? 2"() -> (w613:errorcluster)
          n294 = call-poly <vilib>:"Write To Spreadsheet File.vi"("transpose? (no:F)"=TRUE ("append to file? (new file:F)"), "format (%.3f)"="%.5e", "2D data"=w608) -> ()  [unwired: 5 in, 1 out]
        }
        frame True {
          (unwired) "\r"
          w624 = "\r"
          w626 = "\r"
          # "Vd Trace"
          # "Find Smallest Vd Value"
          # "Picks linear Id based on Smallest Vd"
          # "Dielectric"
          # "Data Values"
          # "Headers"
          n295 = call "HP415xA Op-Download Trace.vi"("error in (no error)"=w725, "trace (variable) name"=w724, "VISA session"=w726) -> ("error out"=w617:errorcluster, "trace"=w723:dbl[])
          n296 = Initialize Array("") -> (w703:string[])  [unwired: 1 in]
          n297 = for {
            N: w730 -> [w734]
            shift-right: [w751] -> w636
            shift-left: w731 -> [w747]
            tunnel: w733 -> [w753]
            tunnel: [w752] -> _ mode=indexing
            shift-right: [w748] -> w631
            shift-left: w732 -> [w750]
            tunnel: [w749] -> w679 mode=indexing
            shift-right: [w744] -> w623
            shift-left: w723 -> [w746]
            tunnel: w719 -> [_]
            tunnel: [w738] -> w680 mode=indexing
            shift-right: [w737] -> w707
            shift-left: w703 -> [w736]
            tunnel: [w734] -> _ mode=indexing
            # "Cuts data at each new loop"
            # "Id Data"
            # "Vd Data"
            # "Vg Data"
            n298 = Search 1D Array(1D array=w747, element=w753, start index (0)=1) -> (index of element=w745:i32)
            n299 = Split 1D Array(array=w746, index=w745) -> (first subarray=w742:dbl[], second subarray=w744:dbl[])
            n300 = Split 1D Array(array=w747, index=w745) -> (first subarray=w752:dbl[], second subarray=w751:dbl[])
            n301 = Split 1D Array(array=w750, index=w745) -> (first subarray=w749:dbl[], second subarray=w748:dbl[])
            n302 = Array Size(array=w742) -> (size(s)=w741:i32)
            n303 = Decrement(x=w741) -> (x-1=w740:i32)
            n304 = Array Subset(array=w742, index=w740) -> (w743:dbl[])  [unwired: 1 in]
            n305 = Number To Exponential String(number=w743) -> (E-format string=w739:string[])  [unwired: 3 in]
            n306 = Build Array (concatenate)("Id", w736) -> (w737:string[])
            n307 = Concatenate Strings(w739) -> (w738:string)
          }
          n308 = call "TempHumSample.vi"("VISA resource name"=refnum<visa-resource-name> "COM4", "error in (no error)"=w617) -> ("CurHum"=w615:dbl, "CurTemp"=w614:dbl)  [unwired: 6 in, 1 out]
          n309 = Fract/Exp String To Number(string=w701) -> (number=w683:dbl)  [unwired: 3 in, 1 out]
          n310 = Fract/Exp String To Number(string=w702) -> (number=w684:dbl)  [unwired: 3 in, 1 out]
          n311 = local read "Temp (K)"() -> (w675:dbl)
          n312 = local read "NumPts"() -> (w682:dbl)
          n313 = local read "NumPts"() -> (w676:dbl)
          n314 = Fract/Exp String To Number(string=w685) -> (number=w677:dbl)  [unwired: 3 in, 1 out]
          n315 = Array Size(array=w623) -> (size(s)=w717:i32)
          n316 = call "STS Calculator.vi"("NumPts"=w676, "Saturation Id"=w631, "Vg Column"=w636) -> ("Sub Threshold Swing"=w669:dbl)  [unwired: 5 in, 3 out]
          n317 = call "Mobility-Vt Calculator_Saturation_12_09_10a_JW.vi"("Vg Column"=w636, "Dielectric Constant"="Dielectric Constant", "Sat Id Column"=w631, "NumPts"=w676, "Length"=w683, "Width"=w684, "Dielectric Thickness"=w677) -> ("Check Cluster"=w665:T8, "Mobility-Sat"=w674:dbl, "VT-Sat"=w670:dbl, "Off I-Sat"=w671:dbl, "On/Off I-Sat"=w672:dbl)  [unwired: 4 out]
          n318 = local write "Check Cluster"(w665) -> ()
          n319 = Decrement(x=w717) -> (x-1=w716:i32)
          n320 = call "Trap Density_VT.vi"("VT"=w670, "Dielectric"=w677) -> ("Trap Density-VT"=w668:dbl)
          n321 = call "Trap Density_STS.vi"("Temp (T) [K]"=w675, "S.T.S. (S)"=w669, "Dielectric"=w677) -> ("Trap Density (N)"=w667:dbl)  [unwired: 8 in]
          n322 = Array Subset(array=w623, index=w716) -> (w715:dbl[])  [unwired: 1 in]
          n323 = Number To Exponential String(number=w715) -> (E-format string=w711:string[])  [unwired: 3 in]
          n324 = Build Array("Sample Temp (K):", "RH (%):", "", "Mobility-Sat (cm^2/Vs):", "Mobility-Lin (cm^2/Vs):", "On/Off I-Sat:", "Off I-Sat (A):", "Vt-Sat (V):", "STS-Sat (V/decade):", "Trap Density-VT (Traps/Vcm^2):", "Trap Density-STS (Traps/Vcm^2):") -> (w699:string[])
          n325 = Build Array (concatenate)(w636, w679, w631) -> (w729:dbl[][])
          n326 = Concatenate Strings(w711) -> (w622:string)
          n327 = Build Array (concatenate)(w680, w622) -> (w678:string[])
          n328 = Fract/Exp String To Number(string=w678) -> (number=w663:dbl[])  [unwired: 3 in, 1 out]
          n329 = Build Array (concatenate)(w679, w631) -> (w661:dbl[][])
          n330 = Build Array("Vg", "Id") -> (w708:string[])
          n331 = Absolute Value(x=w663) -> (abs(x)=w664:dbl[])
          n332 = Insert Into Array(array=w708, index=2, new element=w707) -> (w706:string[])
          n333 = Array Max & Min(array=w664) -> (min index (indices)=w660:i32)  [unwired: 3 out]
          n334 = Index Array(array=w663, index=w660) -> (element=w662:dbl)
          n335 = Transpose 2D Array(2D array=w729) -> (transposed array=w727:dbl[][])
          n336 = Build Array (concatenate)("Vd=", w680, w622) -> (w714:string[])
          n337 = Index Array(array=w661, index (row)=w660) -> (element=w633:dbl[])  [unwired: 1 in]
          n338 = call "Mobility-Vt Calculator_Linear.vi"("Vg Column"=w636, "Vd"=w662, "Lin Id Column"=w633, "NumPts"=w682, "Length"=w683, "Width"=w684, "Dielectric Thickness"=w677, "Dielectric Constant"="Dielectric Constant") -> ("Mobility-Lin"=w673:dbl)  [unwired: 1 in, 6 out]
          n339 = Build Array(w614, w615, w674, w673, w672, w671, w670, w669, w668, w667) -> (w698:dbl[])
          n340 = Number To Exponential String(number=w698) -> (E-format string=w658:string[])  [unwired: 3 in]
          n341 = Bundle("Mobility-Sat"=w674, "Mobility-Lin"=w673, "On/Off I-Sat"=w672, "Off I-Sat"=w671, "VT-Sat"=w670, "Sub Threshold Swing"=w669, "Trap Density-VT"=w668, "Trap Density (N)"=w667) -> (w666:T9)  [unwired: 1 in]
          n342 = local write "Output"(w666) -> ()
          n343 = Insert Into Array(array=w658, index=1, new element="") -> (w655:string[])
          n344 = Build Array(w699, w655) -> (w654:string[][])
          n345 = Transpose 2D Array(2D array=w654) -> (transposed array=w653:string[][])
          n346 = Array To Spreadsheet String(array=w714, 3:"%s") -> (spreadsheet string=w718:string)  [unwired: 1 in]
          n347 = Array To Spreadsheet String(array=w706, 3:"%s") -> (spreadsheet string=w712:string)  [unwired: 1 in]
          n348 = Array To Spreadsheet String(array=w653, 3:"%s") -> (spreadsheet string=w696:string)  [unwired: 1 in]
          n349 = Array To Spreadsheet String(array=w727, 3:"%.5e" ("format string")) -> (spreadsheet string=w720:string)  [unwired: 1 in]
          n350 = Concatenate Strings(w627, w626, w619, w626, w625, w696, w626, w718, w712, w720, w624) -> (w722:string)
          n351 = Absolute Value(x=w633) -> (abs(x)=w638:dbl[])
          n352 = Absolute Value(x=w631) -> (abs(x)=w635:dbl[])
          n353 = Absolute Value(x=w633) -> (abs(x)=w632:dbl[])
          n354 = Absolute Value(x=w631) -> (abs(x)=w630:dbl[])
          n355 = Square Root(x=w638) -> (sqrt(x)=w637:dbl[])
          n356 = Square Root(x=w635) -> (sqrt(x)=w634:dbl[])
          n357 = Concatenate Strings(w627, w626, w619, w624, w625, w624) -> (w621:string)
          n358 = Bundle("trace"=w636, w632) -> (w641:cluster{"trace":dbl[], dbl[]})  [unwired: 1 in]
          n359 = Bundle("trace"=w636, w630) -> (w644:cluster{"trace":dbl[], dbl[]})  [unwired: 1 in]
          n360 = Bundle("trace"=w636, w637) -> (w640:cluster{"trace":dbl[], dbl[]})  [unwired: 1 in]
          n361 = Bundle("trace"=w636, w634) -> (w645:cluster{"trace":dbl[], dbl[]})  [unwired: 1 in]
          n362 = Bundle("trace"=w636, w633) -> (w647:cluster{"trace":dbl[], dbl[]})  [unwired: 1 in]
          n363 = Bundle("trace"=w636, "trace"=w631) -> (w649:cluster{"trace":dbl[], "trace":dbl[]})  [unwired: 1 in]
          n364 = Build Array(w640) -> (w639:cluster{"trace":dbl[], dbl[]}[])
          n365 = Build Array(w641) -> (w629:cluster{"trace":dbl[], dbl[]}[])
          n366 = Build Array(w645) -> (w642:cluster{"trace":dbl[], dbl[]}[])
          n367 = Build Array(w644) -> (w643:cluster{"trace":dbl[], dbl[]}[])
          n368 = Build Array(w647) -> (w646:cluster{"trace":dbl[], dbl[]}[])
          n369 = Build Array(w649) -> (w648:cluster{"trace":dbl[], "trace":dbl[]}[])
          n370 = local read "Graph Cluster"() -> (w651:T1)
          n371 = local read "Input Path"() -> (w686:path)
          n372 = Bundle By Name(cluster=w651, "Linear Sqrt"=w639, "Linear Log"=w629, "Linear Raw"=w646, "Saturation Sqrt"=w642, "Saturation Log"=w643, "Saturation Raw"=w648, "Gate Current"=w628) -> (w650:T1)
          n373 = call <vilib>:"Write Characters To File.vi"("append to file? (new file:F)"=TRUE, "character string"=w722, "file path (dialog if empty)"=w686) -> ("new file path (Not A Path if cancelled)"=w694:path)  [unwired: 2 in]
          n374 = local write "Graph Cluster"(w650) -> ()
          n375 = local write "Output Path"(w694) -> ()
        }
      }
      n376 = case shown="True" w579 {
        tunnel: w563 -> [_ w763]
        tunnel: w556 -> [_ w764]
        tunnel: w577 -> [_ w762]
        tunnel: w571 -> [_ w761]
        tunnel: w578 -> [_ w760]
        tunnel: w575 -> [_ w759]
        tunnel: w560 -> [_ w758]
        tunnel: w555 -> [_ w757]
        tunnel: w554 -> [_ w756]
        tunnel: w553 -> [_ w755]
        frame False {
        }
        frame True {
          n377 = case shown="True" w764 {
            tunnel: w763 -> [_ w793]
            tunnel: w762 -> [w768 w805]
            tunnel: w761 -> [_ w804]
            tunnel: w760 -> [w769 w803]
            tunnel: w759 -> [_ w802]
            tunnel: w758 -> [_ w790]
            tunnel: w757 -> [_ w783]
            tunnel: w756 -> [_ w782]
            tunnel: w755 -> [_ w771]
            frame False {
              n378 = Build Array(w768, w769) -> (w767:dbl[][])
              n379 = call-poly <vilib>:"Write To Spreadsheet File.vi"("transpose? (no:F)"=TRUE, "format (%.3f)"="%.5e", "2D data"=w767) -> ()  [unwired: 5 in, 1 out]
            }
            frame True {
              n380 = for {
                N: w793 -> [_]
                shift-right: [w819] -> w801
                shift-left: w805 -> [w820]
                tunnel: w804 -> [w822]
                tunnel: [w818] -> _ mode=indexing
                shift-right: [w815] -> w785
                shift-left: w803 -> [w817]
                tunnel: [w816] -> w800 mode=indexing
                shift-right: [w812] -> w797
                shift-left: w802 -> [w813]
                tunnel: [w809] -> w794 mode=indexing
                shift-right: [w808] -> w784
                shift-left: _ -> [w807]
                tunnel: w783 -> [w806]
                n381 = Search 1D Array(1D array=w820, element=w822, start index (0)=1) -> (index of element=w814:i32)
                n382 = Split 1D Array(array=w820, index=w814) -> (first subarray=w818:dbl[], second subarray=w819:dbl[])
                n383 = Split 1D Array(array=w817, index=w814) -> (first subarray=w816:dbl[], second subarray=w815:dbl[])
                n384 = Split 1D Array(array=w813, index=w814) -> (first subarray=w810:dbl[], second subarray=w812:dbl[])
                n385 = Index Array(array=w810, index=1) -> (element=w809:dbl)
                n386 = Build Array (concatenate)(w806, w807) -> (w808:string[])
              }
              n387 = Build Array (concatenate)(w801, w800, w785) -> (w799:dbl[][])
              n388 = Index Array(array=w797, index=1) -> (element=w795:dbl)
              n389 = Transpose 2D Array(2D array=w799) -> (transposed array=w798:dbl[][])
              n390 = Insert Into Array(array=w794, index=w793, new element=w795) -> (w792:dbl[])
              n391 = Array To Spreadsheet String(array=w792, 3:"%.5e" ("format string")) -> (spreadsheet string=w779:string)  [unwired: 1 in]
              n392 = Concatenate Strings(w790, "= " ("string")) -> (w780:string)
              n393 = Array To Spreadsheet String(array=w798, 3:"%.5e" ("format string")) -> (spreadsheet string=w777:string)  [unwired: 1 in]
              n394 = Build Array(w782, w783) -> (w787:string[])
              n395 = Insert Into Array(array=w787, index=2, new element=w784) -> (w786:string[])
              n396 = Concatenate Strings(w780, w779) -> (w778:string)
              n397 = Array To Spreadsheet String(array=w786, 3:"%s") -> (spreadsheet string=w776:string)  [unwired: 1 in]
              n398 = Concatenate Strings(w778, w776, w777) -> (w770:string)
              "concatenated string" <- w770
              n399 = Concatenate Strings(w771, w770) -> (w773:string)
              n400 = local read "LKG Path"() -> (w772:path)
              n401 = call <vilib>:"Write Characters To File.vi"("append to file? (new file:F)"=TRUE, "character string"=w773, "file path (dialog if empty)"=w772) -> ()  [unwired: 2 in, 1 out]
            }
          }
        }
      }
      n402 = call "HP415xA Sys-Error Query.vi"("VISA session"=w572, "error in (no error)"=w576) -> ("error out"=w604:errorcluster)  [unwired: 2 in, 1 out]
      n403 = call "HP415xA  Close.vi"("error in (no error)"=w604, "VISA session"=w572) -> ("error out"=w605:errorcluster)
      n404 = local write "error?"(w605) -> ()
    }
  }
